vi "Comic Manager.vi"() -> ()   [LabVIEW 2024]
uses:
  TypeDefs/comic--cluster.ctl
  TypeDefs/series--cluster.ctl
  <userlib>/_OpenG.lib/file/file.llb/Strip Path Extension - String__ogtk.vi
  <userlib>/_OpenG.lib/file/file.llb/Strip Path Extension - Path__ogtk.vi
  <userlib>/_OpenG.lib/array/array.llb/Remove Duplicates from 1D Array (DBL)__ogtk.vi
  <userlib>/_OpenG.lib/array/array.llb/Sort 1D Array (String)__ogtk.vi
  <userlib>/_OpenG.lib/array/array.llb/openg_array.lvlib
  <userlib>/_OpenG.lib/file/file.llb/openg_file.lvlib
  <vilib>/httpClient/LabVIEWHTTPClient.lvlib
  <vilib>/addons/_JKI.lib/Serialization/JSON/JKI JSON Serialization.lvlib
panel:
  out "More Avail":bool
  out "Available?":bool
  in  "series tabs":enum32{"Add Issues", "Edit Series"}(tab)
  in  "New Issues":i32(listbox)
  out "new issue cover":picture
  in  "New Comics":path=path "D:/Comics/To Be Filed/Marvel"
  in  "move selected new":bool
  in  "move all new":bool
  in  "refresh":bool
  out "matching count":bool
  in  "comic info":T1
  in  "apply series changes":bool
  in  "series info":T2
  in  "Marvel Issues":i32(listbox)
  in  "launch renamer":bool
  in  "filter string":string
  in  "rename all cbz":bool
  in  "rename selected clz":bool
  in  "delete json issue":bool
  in  "rename json issue":bool
  out "synced":bool
  in  "create new folder":bool
  in  "json file path":path
  out "current details":i32(listbox)
  out "json details":i32(listbox)
  in  "launch cleaner":bool
  in  "Filter Current":bool
  out "json issue cover":picture
  out "current issue cover":picture
  in  "Series":i32(listbox)
  in  "Collected Issues":i32(listbox)
  in  "Folder":i32(listbox)
  in  "exit":bool
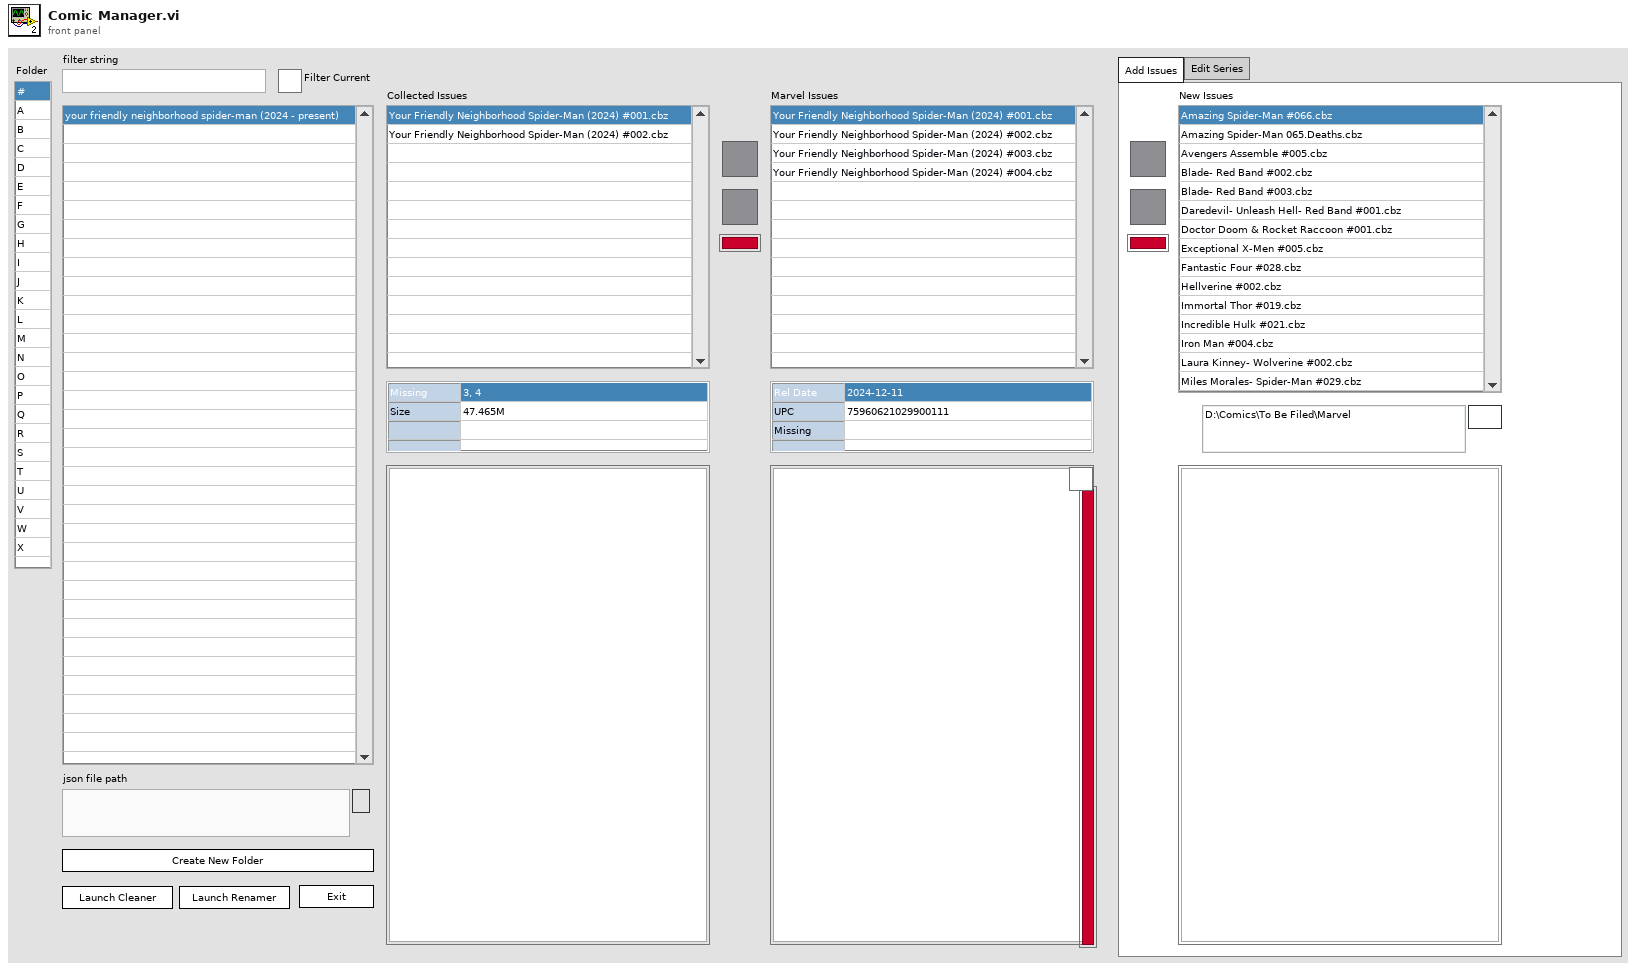
[diagram p1: front panel]
types:
  T1 = cluster{"rel date":string, "title":string, "description":string, "creators":string[], "characters":string[]}
  T2 = cluster{"seriesType":string, "title":string, "id":u32, "description":string, "start year":u32, "end year":u32, "tags":string[]}
  T3 = enum32{"Invalid", "Standard", "Closed", "Hidden", "Minimized", "Maximized"}
  T4 = enum32{"invalid app kind", "Development System", "Run Time System", "Student Edition", "Embedded LabVIEW", "Evaluation", "Custom"}
  T5 = enum16{"open", "replace", "create", "open or create", "replace or create", "replace or create with confirmation"}
  T6 = typedef "comic--cluster.ctl" = cluster{"id":i32, "digitalId":i32, "title":string, "issueNumber":i32, "variantDescription":string, "description":string, "modified":variant, "upc":string, "format":string, "pageCount":i32, "resourceURI":string, "urls":cluster{"type":string, "url":string}[], "series":cluster{"resourceURI":string, "name":string}, "dates":cluster{"type":string, "date":string}[], "prices":cluster{"price":dbl, "type":string}[], "thumbnail":cluster{"path":string, "extension":string}, "images":cluster{"path":string, "extension":string}[], "creators":cluster{"available":i32, "returned":i32, "collectionURI":string, "items":cluster{"resourceURI":string, "name":string, "role":string}[]}, "characters":cluster{"available":i32, "returned":i32, "collectionURI":string, "items":cluster{"resourceURI":string, "name":string}[]}, "stories":cluster{"available":i32, "returned":i32, "collectionURI":string, "items":cluster{"resourceURI":string, "name":string, "type":string}[]}, "events":cluster{"available":i32, "returned":i32, "collectionURI":string, "items":cluster{"resourceURI":string, "name":string}[]}}
  T7 = typedef "series--cluster.ctl" = cluster{"id":i32, "title":string, "description":string, "resourceURI":string, "urls":cluster{"type":string, "url":string}[], "startYear":i32, "endYear":i32, "rating":string, "type":string, "modified":variant, "thumbnail":cluster{"path":string, "extension":string}, "creators":cluster{"available":i32, "returned":i32, "collectionURI":string, "items":cluster{"resourceURI":string, "name":string, "role":string}[]}, "comics":cluster{"available":i32, "returned":i32, "collectionURI":string, "items":cluster{"resourceURI":string, "name":string}[]}, "characters":cluster{"available":i32, "returned":i32, "collectionURI":string, "items":cluster{"resourceURI":string, "name":string}[]}, "stories":cluster{"available":i32, "returned":i32, "collectionURI":string, "items":cluster{"resourceURI":string, "name":string, "type":string}[]}, "events":cluster{"available":i32, "returned":i32, "collectionURI":string, "items":cluster{"resourceURI":string, "name":string}[]}, "next":variant, "previous":variant, "tags":string[]}
  T8 = cluster{"Core":cluster{"Current VI Reference":refnum<vi>, "Close Panel on Exit?":bool}, "repo path":path, "series path":path, "json present":bool, "comic jsons":T6[], "local working folder":path, "display web":bool, "new working folder":path, "current missing":string, "json missing":string, "json dup":string, "current size":string, "web cover path":path, "series json":T7}
  T9 = cluster{"Current VI Reference":refnum<vi>, "Close Panel on Exit?":bool}
  T10 = typedef "comics.reply--cluster.ctl" = cluster{"code":i32, "status":string, "etag":string, "data":cluster{"offset":i32, "limit":i32, "total":i32, "count":i32, "results":T6[]}}
  T11 = typedef "imagedata.ctl" = cluster{"image type":i32, "image depth":i32, "image":u8[], "mask":u8[], "colors":u32[], "Rectangle":cluster{"left":i16, "top":i16, "right":i16, "bottom":i16}}
  T12 = typedef "LVBoundsTypeDef.ctl" = cluster{"Width":u32, "Height":u32}
  T13 = cluster{"resourceURI":string, "name":string, "role":string}[]
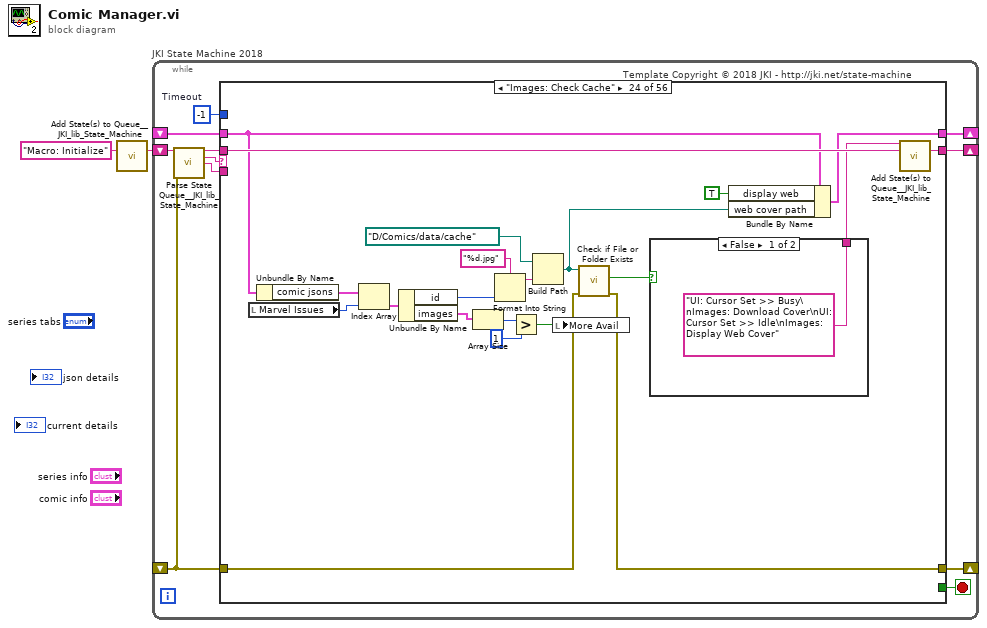
[diagram p0: block diagram]
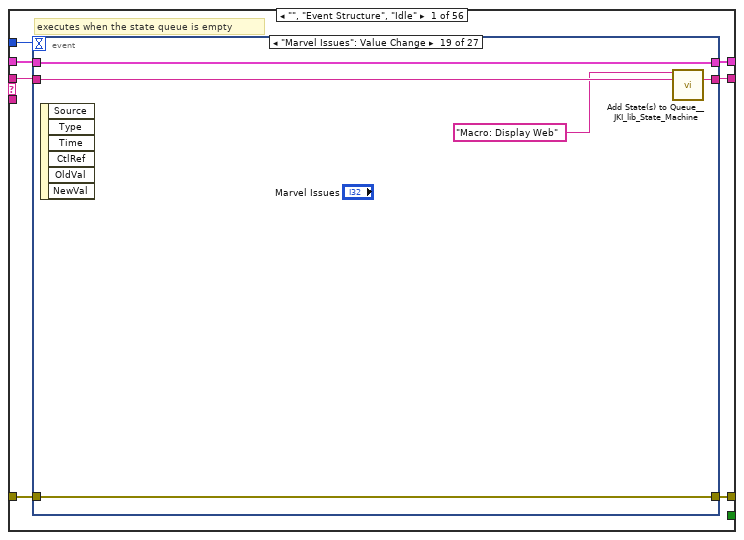
[diagram p2: hidden frame]
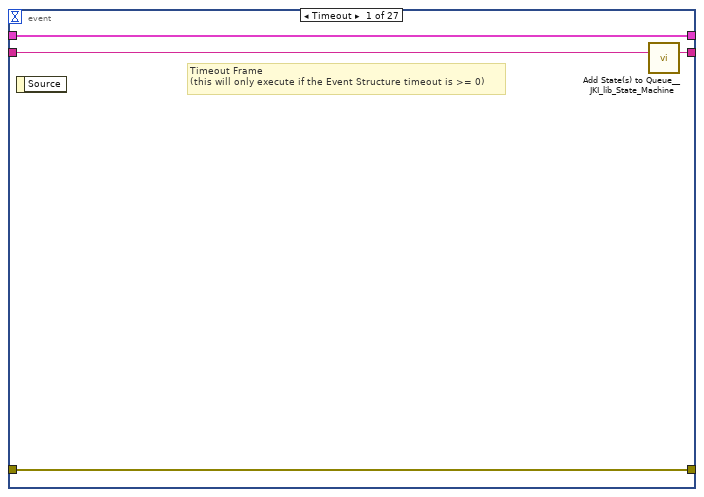
[diagram p3: hidden frame]
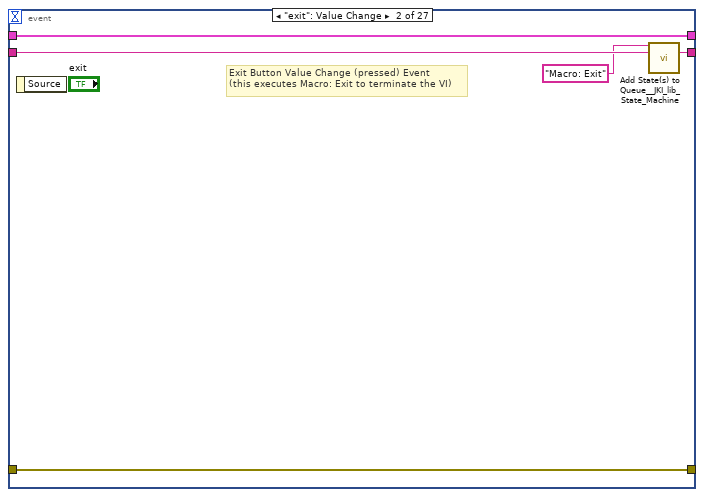
[diagram p4: hidden frame]
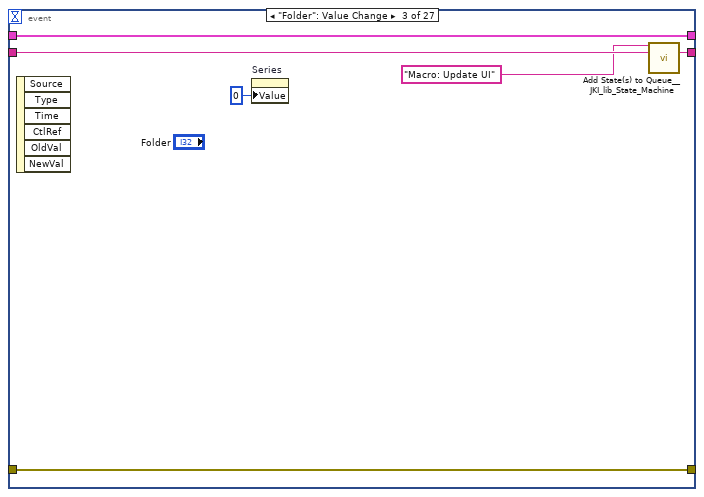
[diagram p5: hidden frame]
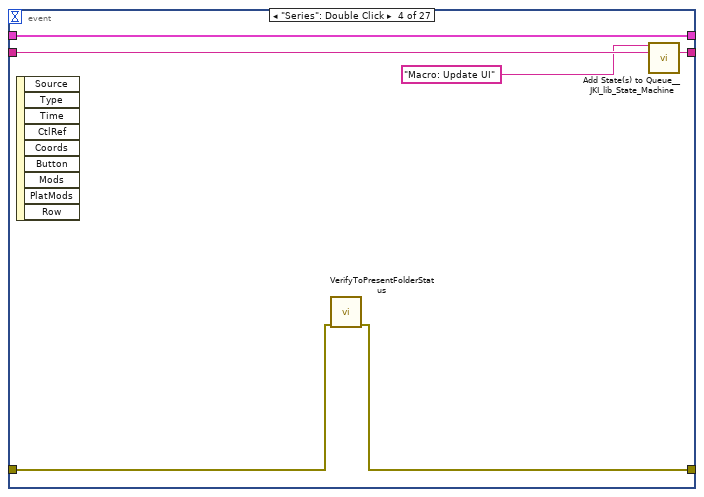
[diagram p6: hidden frame]
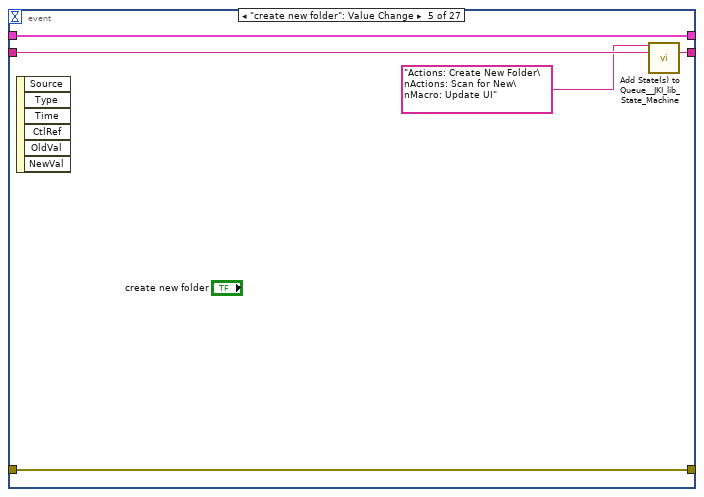
[diagram p7: hidden frame]
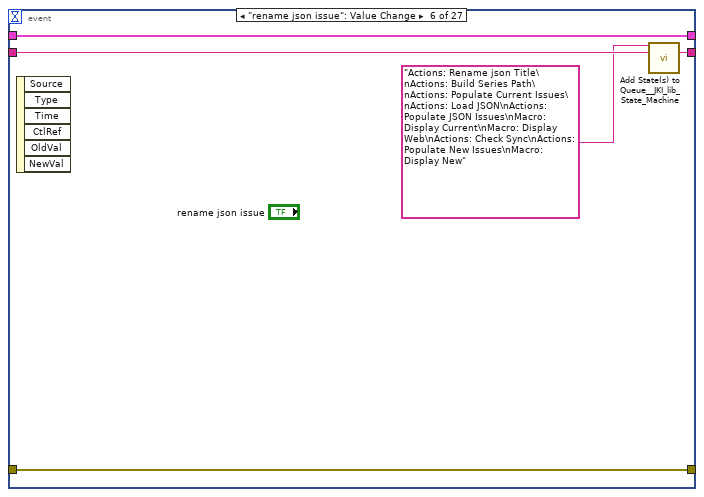
[diagram p8: hidden frame]
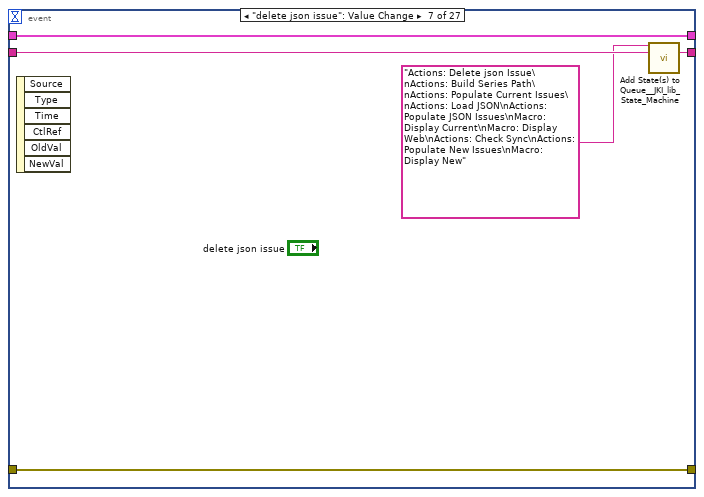
[diagram p9: hidden frame]
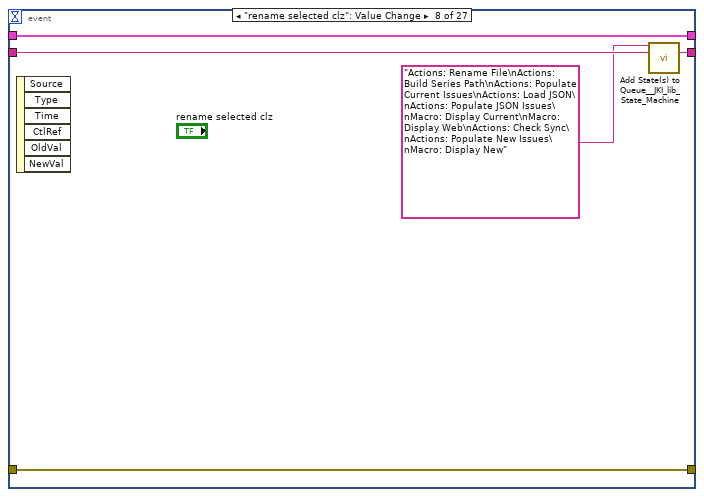
[diagram p10: hidden frame]
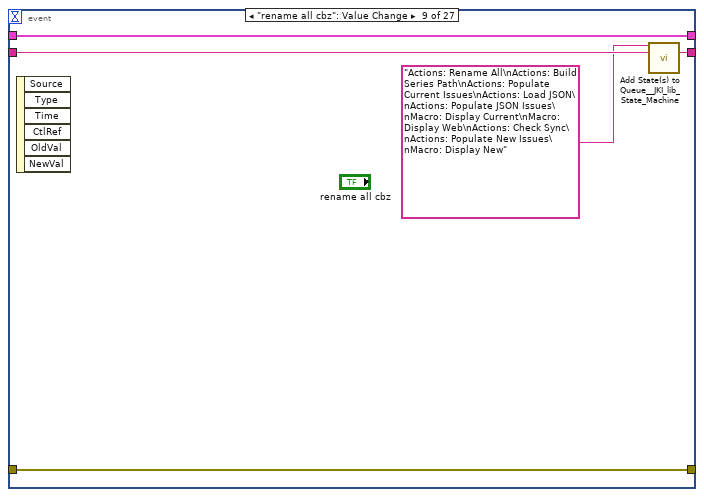
[diagram p11: hidden frame]
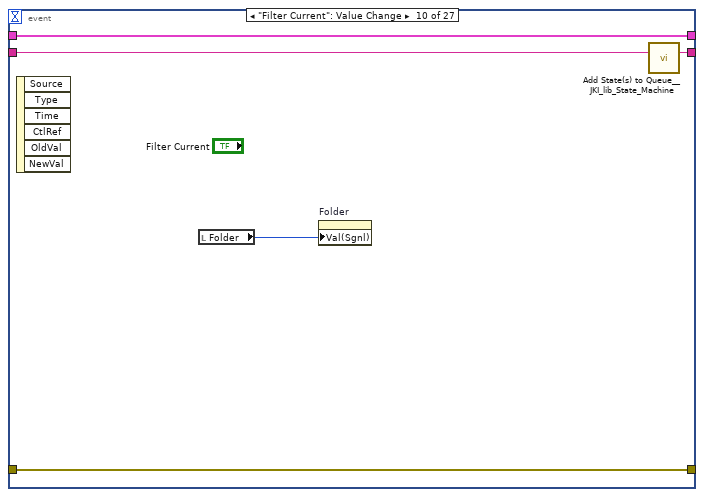
[diagram p12: hidden frame]
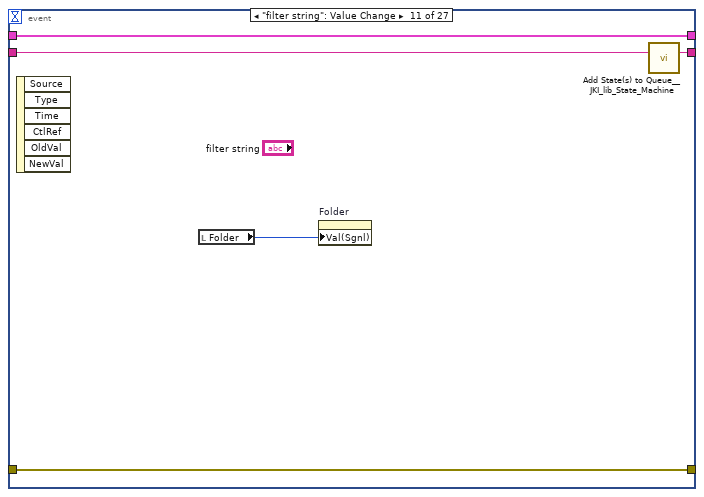
[diagram p13: hidden frame]
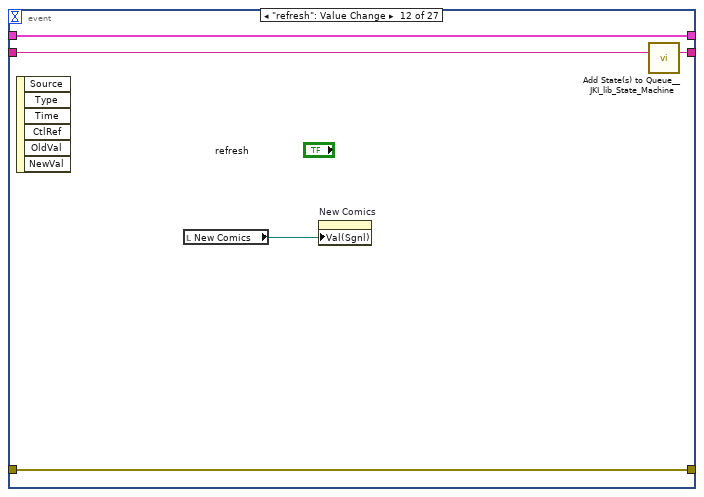
[diagram p14: hidden frame]
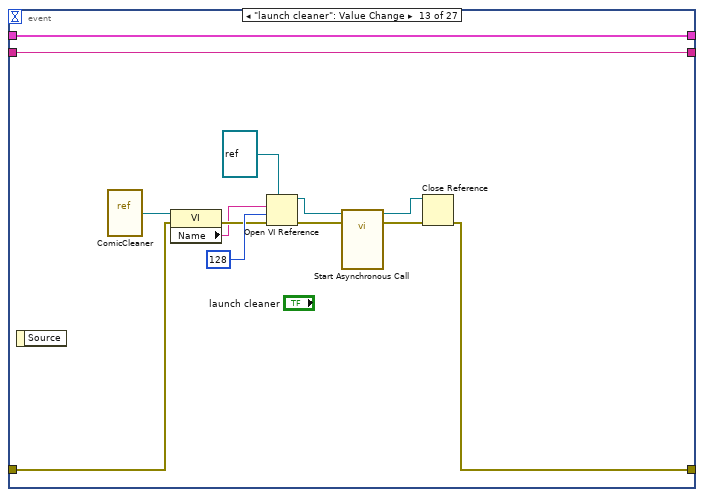
[diagram p15: hidden frame]
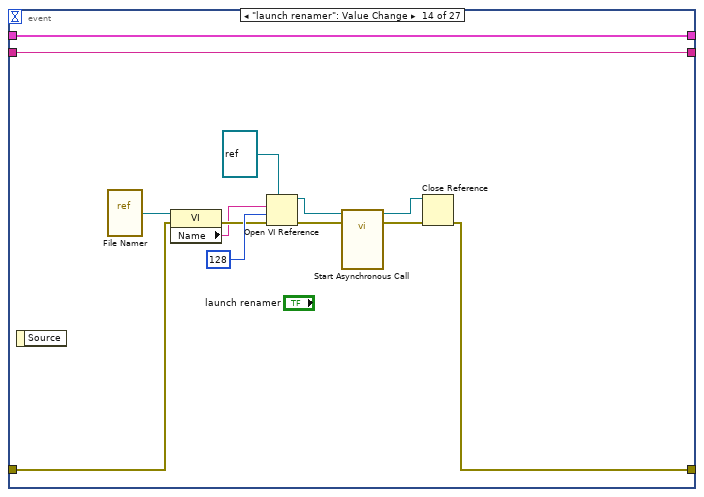
[diagram p16: hidden frame]
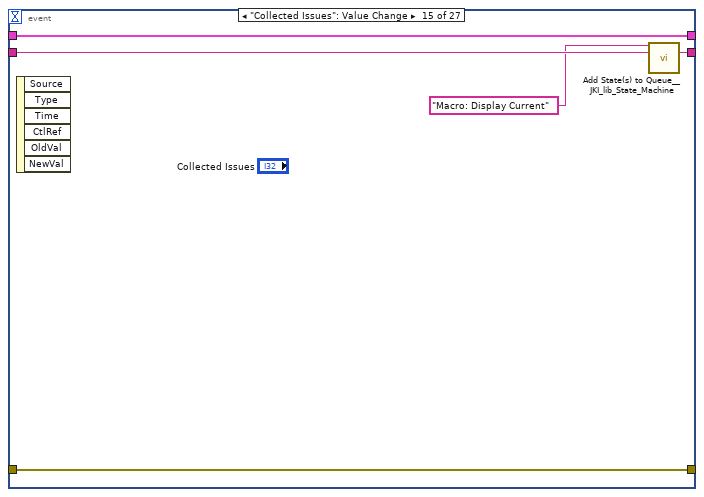
[diagram p17: hidden frame]
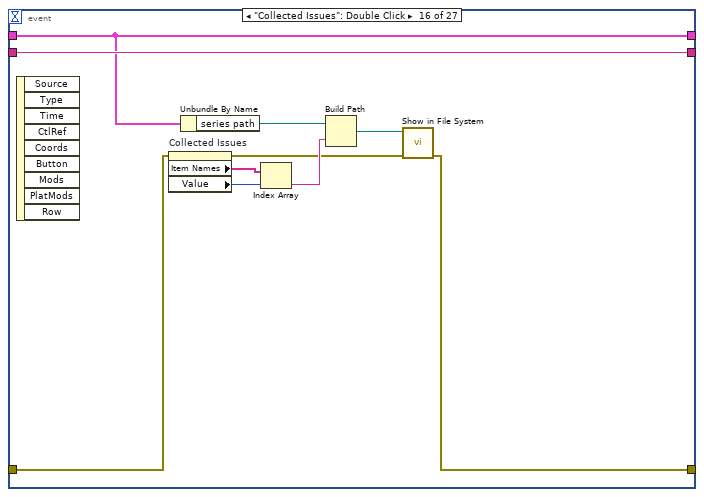
[diagram p18: hidden frame]
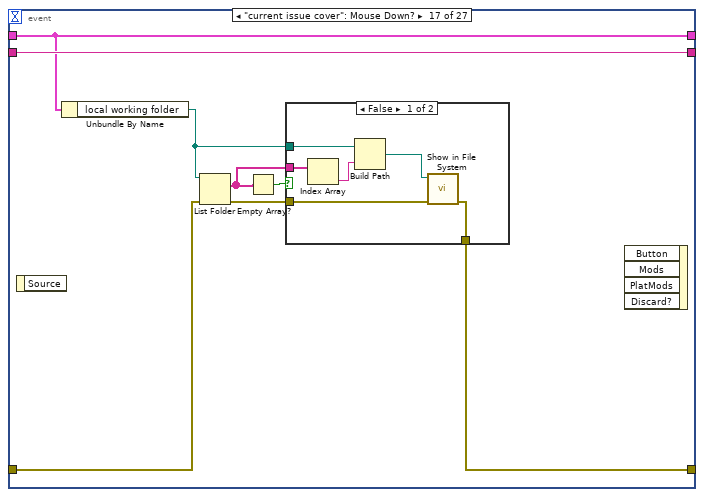
[diagram p19: hidden frame]
diagram:
  n1 = call <vilib>:"Add State(s) to Queue__JKI_lib_State_Machine.vi"("State(s) in (\"\")"="Macro: Initialize") -> ("States Out"=w2:string)  [unwired: 14 in]
  n2 = while "JKI State Machine 2018" {
    shift-right: [w6] -> _
    shift-left: _ -> [w5]
    shift-right: [w9] -> _
    shift-left: _ -> [w3]
    shift-right: [w8] -> _
    shift-left: w2 -> [w10]
    stop <- w7 stop-if-true
    w4 = -1  # Timeout
    # "Template Copyright © 2018 JKI - http://jki.net/state-machine"
    n3 = call <vilib>:"Parse State Queue__JKI_lib_State_Machine.vi"("State Queue"=w10, "Error In (no error)"=w3) -> ("Remaining States"=w12:string, "Current State"=w13:string, "Arguments"=w11:string)  [unwired: 11 in]
    n4 = case shown="\"Images: Check Cache\"" w13 {
      selector: w13 -> [_ _ w205 _ _ _ _ _ _ _ _ _ _ _ _ _ _ _ _ _ _ _ _ _ _ _ _ _ _ _ _ _ _ _ _ _ _ _ _ _ _ _ _ _ _ _ _ _ _ _ _ _ _ _ _ _]
      tunnel: w12 -> [w20 w204 w209 w228 w234 w239 w243 w261 w282 w300 w304 w314 w320 w331 w400 w405 w410 w415 w420 w425 w430 w440 w444 w465 w483 w514 w533 w562 w568 w592 w627 w651 w691 w727 w731 w748 w765 w792 w799 w821 w849 w857 w895 w930 w956 w979 w1016 w1034 w1064 w1082 w1108 w1135 w1145 w1155 w1165 w1210]
      tunnel: w11 -> [_ _ _ _ _ _ _ _ _ _ _ _ w315 w325 _ _ _ _ _ _ _ _ _ _ _ _ _ _ _ _ _ _ _ _ _ _ _ _ _ _ _ _ _ _ _ _ _ _ _ _ _ _ _ _ _ _]
      tunnel: w5 -> [w18 w201 w207 w221 w231 w237 w240 _ w272 w295 w301 w312 w318 w327 w397 w402 w407 w412 w417 w422 w427 w437 w441 w449 w471 w512 w523 w559 w565 w583 w618 w645 w682 w712 w728 w744 w762 w782 w797 w819 w847 w855 w893 w928 w954 w969 w1012 w1032 w1056 w1077 w1095 w1121 w1143 w1153 w1161 w1206]
      tunnel: [w17 w202 w211 w225 errorcluster {"status"=FALSE, "code"=0, "source"=""} ("error out") w236 w241 w258 w273 w296 w302 w306 w316 w328 w398 w403 w408 w413 w418 w423 w428 w438 w442 w455 w468 w488 w524 w558 w564 w569 w605 w649 w684 w711 w729 w741 w763 w766 w794 w816 w846 w851 w892 w925 w944 w961 w1006 w1031 w1049 w1074 w1100 w1123 w1137 w1148 w1157 w1182] -> w9
      tunnel: w3 -> [w16 w202 w210 w225 w230 w236 w241 w258 w266 w297 w302 w311 w317 w329 w398 w403 w408 w413 w418 w423 w428 w438 w442 w456 w473 w497 w525 w557 w563 w582 w617 w644 w683 w710 w729 w741 w763 w779 w795 w817 w845 w852 w889 w926 w945 w964 w995 w1030 w1050 w1075 w1102 w1124 w1141 w1152 w1158 w1208]
      tunnel: [w19 w203 w208 w227 w233 w238 w242 w260 w281 w299 w303 w313 w319 w330 w399 w404 w409 w414 w419 w424 w429 w439 w443 w464 w482 w513 w532 w561 w567 w591 w626 w650 w690 w726 w730 w747 w764 w791 w798 w820 w848 w856 w894 w929 w955 w978 w1015 w1033 w1063 w1081 w1107 w1134 w1144 w1154 w1164 w1209] -> w8
      tunnel: [_ _ _ _ _ TRUE _ _ _ _ _ _ _ _ _ _ _ _ _ _ _ _ _ _ _ _ _ _ _ _ _ _ _ _ _ _ _ _ _ _ _ _ _ _ _ _ _ _ _ _ _ _ _ _ _ _] -> w7
      tunnel: [w15 w201 w207 w226 w231 w237 w240 w259 w271 w295 w301 w312 w318 w327 w397 w402 w407 w412 w417 w422 w427 w437 w441 w451 w471 w511 w522 w559 w565 w583 w618 w645 w680 w712 w728 w744 w762 w781 w797 w819 w847 w850 w891 w928 w954 w965 w1012 w1032 w1056 w1077 w1095 w1120 w1143 w1153 w1160 w1205] -> w6
      tunnel: w4 -> [w14 _ _ _ _ _ _ _ _ _ _ _ _ _ _ _ _ _ _ _ _ _ _ _ _ _ _ _ _ _ _ _ _ _ _ _ _ _ _ _ _ _ _ _ _ _ _ _ _ _ _ _ _ _ _ _]
      frame "", "Event Structure", "Idle" {
        # "executes when the state queue is empty"
        n5 = event shown="[18] \"Marvel Issues\": Value Change" {
          selector: _ -> [_ _ _ _ _ _ _ _ _ _ _ _ _ _ _ _ _ _ _ _ _ _ _ _ _ _ _]
          dyn-events: _ -> [_ _ _ _ _ _ _ _ _ _ _ _ _ _ _ _ _ _ _ _ _ _ _ _ _ _ _]
          timeout: w14 -> [_ _ _ _ _ _ _ _ _ _ _ _ _ _ _ _ _ _ _ _ _ _ _ _ _ _ _]
          tunnel: w20 -> [w24 w29 w35 w41 w46 w51 w56 w61 w66 w71 w76 w81 w93 w106 w112 w122 w130 w144 w157 w161 w169 w174 w179 w184 w188 w194 w200]
          tunnel: [w23 w28 w34 w40 w45 w50 w55 w60 w65 w70 w75 w80 w93 w106 w111 w122 w130 w144 w156 w163 w168 w173 w178 w183 w186 w193 w199] -> w19
          tunnel: w18 -> [w21 w26 w32 w39 w43 w48 w53 w58 w63 w68 w73 w78 w94 w107 w109 w121 w129 w145 w154 w160 w166 w171 w176 w182 w189 w191 w197]
          tunnel: [w22 w27 w33 w36 w44 w49 w54 w59 w64 w69 w74 w79 w87 w100 w110 w114 w125 w140 w155 w159 w167 w172 w177 w181 w185 w190 w198] -> w17
          tunnel: w16 -> [w22 w27 w33 w37 w44 w49 w54 w59 w64 w69 w74 w79 w86 w99 w110 w115 w127 w143 w155 w159 w167 w172 w177 w181 w185 w190 w198]
          tunnel: [w21 w26 w32 w39 w43 w48 w53 w58 w63 w68 w73 w78 w94 w107 w109 w121 w129 w145 w154 w160 w166 w171 w176 w182 w189 w191 w197] -> w15
          event Timeout {
            # "Timeout Frame\n(this will only execute if the Event Structure timeout is >= 0)"
            n6 = event-data() -> ()  [unwired: 1 in, 1 out]
            n7 = call <vilib>:"Add State(s) to Queue__JKI_lib_State_Machine.vi"("State(s) in (\"\")"=w24) -> ("States Out"=w23:string)  [unwired: 14 in]
          }
          event "exit": Value Change {
            # "Exit Button Value Change (pressed) Event\n(this executes Macro: Exit to terminate the VI)"
            n8 = event-data() -> ()  [unwired: 1 in, 1 out]
            n9 = call <vilib>:"Add State(s) to Queue__JKI_lib_State_Machine.vi"("State(s) in Front (\"\")"="Macro: Exit", "State(s) in (\"\")"=w29) -> ("States Out"=w28:string)  [unwired: 13 in]
          }
          event "Folder": Value Change {
            n10 = event-data() -> ()  [unwired: 1 in, 6 out]
            n11 = property on="Series" class="LstBox (strict)"("Value"=0 ("Series")) -> ()  [unwired: 2 in, 2 out]
            n12 = call <vilib>:"Add State(s) to Queue__JKI_lib_State_Machine.vi"("State(s) in Front (\"\")"="Macro: Update UI", "State(s) in (\"\")"=w35) -> ("States Out"=w34:string)  [unwired: 13 in]
          }
          event "Series": Double Click {
            n13 = event-data() -> ()  [unwired: 1 in, 9 out]
            n14 = call "VerifyToPresentFolderStatus.vi"("error in (no error)"=w37) -> ("error out"=w36:errorcluster)  [unwired: 9 in, 1 out]
            n15 = call <vilib>:"Add State(s) to Queue__JKI_lib_State_Machine.vi"("State(s) in Front (\"\")"="Macro: Update UI", "State(s) in (\"\")"=w41) -> ("States Out"=w40:string)  [unwired: 13 in]
          }
          event "create new folder": Value Change {
            n16 = event-data() -> ()  [unwired: 1 in, 6 out]
            n17 = call <vilib>:"Add State(s) to Queue__JKI_lib_State_Machine.vi"("State(s) in Front (\"\")"="Actions: Create New Folder\nActions: Scan for New\nMacro: Update UI", "State(s) in (\"\")"=w46) -> ("States Out"=w45:string)  [unwired: 13 in]
          }
          event "rename json issue": Value Change {
            n18 = event-data() -> ()  [unwired: 1 in, 6 out]
            n19 = call <vilib>:"Add State(s) to Queue__JKI_lib_State_Machine.vi"("State(s) in Front (\"\")"="Actions: Rename json Title\nActions: Build Series Path\nActions: Populate Current Issues\nActions: Load JSON\nActions: Populate JSON Issues\nMacro: Display Current\nMacro: Display Web\nActions: Check Sync\nActions: Populate New Issues\nMacro: Display New", "State(s) in (\"\")"=w51) -> ("States Out"=w50:string)  [unwired: 13 in]
          }
          event "delete json issue": Value Change {
            n20 = event-data() -> ()  [unwired: 1 in, 6 out]
            n21 = call <vilib>:"Add State(s) to Queue__JKI_lib_State_Machine.vi"("State(s) in Front (\"\")"="Actions: Delete json Issue\nActions: Build Series Path\nActions: Populate Current Issues\nActions: Load JSON\nActions: Populate JSON Issues\nMacro: Display Current\nMacro: Display Web\nActions: Check Sync\nActions: Populate New Issues\nMacro: Display New", "State(s) in (\"\")"=w56) -> ("States Out"=w55:string)  [unwired: 13 in]
          }
          event "rename selected clz": Value Change {
            n22 = event-data() -> ()  [unwired: 1 in, 6 out]
            n23 = call <vilib>:"Add State(s) to Queue__JKI_lib_State_Machine.vi"("State(s) in Front (\"\")"="Actions: Rename File\nActions: Build Series Path\nActions: Populate Current Issues\nActions: Load JSON\nActions: Populate JSON Issues\nMacro: Display Current\nMacro: Display Web\nActions: Check Sync\nActions: Populate New Issues\nMacro: Display New", "State(s) in (\"\")"=w61) -> ("States Out"=w60:string)  [unwired: 13 in]
          }
          event "rename all cbz": Value Change {
            n24 = event-data() -> ()  [unwired: 1 in, 6 out]
            n25 = call <vilib>:"Add State(s) to Queue__JKI_lib_State_Machine.vi"("State(s) in Front (\"\")"="Actions: Rename All\nActions: Build Series Path\nActions: Populate Current Issues\nActions: Load JSON\nActions: Populate JSON Issues\nMacro: Display Current\nMacro: Display Web\nActions: Check Sync\nActions: Populate New Issues\nMacro: Display New", "State(s) in (\"\")"=w66) -> ("States Out"=w65:string)  [unwired: 13 in]
          }
          event "Filter Current": Value Change {
            n26 = event-data() -> ()  [unwired: 1 in, 6 out]
            n27 = local read "Folder"() -> (w67:i32)
            n28 = property on="Folder" class="LstBox (strict)"("Val(Sgnl)"=w67) -> ()  [unwired: 2 in, 2 out]
            n29 = call <vilib>:"Add State(s) to Queue__JKI_lib_State_Machine.vi"("State(s) in (\"\")"=w71) -> ("States Out"=w70:string)  [unwired: 14 in]
          }
          event "filter string": Value Change {
            n30 = event-data() -> ()  [unwired: 1 in, 6 out]
            n31 = local read "Folder"() -> (w72:i32)
            n32 = property on="Folder" class="LstBox (strict)"("Val(Sgnl)"=w72) -> ()  [unwired: 2 in, 2 out]
            n33 = call <vilib>:"Add State(s) to Queue__JKI_lib_State_Machine.vi"("State(s) in (\"\")"=w76) -> ("States Out"=w75:string)  [unwired: 14 in]
          }
          event "refresh": Value Change {
            n34 = event-data() -> ()  [unwired: 1 in, 6 out]
            n35 = local read "New Comics"() -> (w77:path)
            n36 = property on="New Comics" class="Path"("Val(Sgnl)"=w77) -> ()  [unwired: 2 in, 2 out]
            n37 = call <vilib>:"Add State(s) to Queue__JKI_lib_State_Machine.vi"("State(s) in (\"\")"=w81) -> ("States Out"=w80:string)  [unwired: 14 in]
          }
          event "launch cleaner": Value Change {
            n38 = event-data() -> ()  [unwired: 1 in, 1 out]
            n39 = vi-ref "ComicCleaner.vi"() -> (w91:refnum<vi>)
            n40 = property class="VI"(reference=w91, error in=w86) -> (error out=w90:errorcluster, "Name"=w89:string)  [unwired: 1 out]
            n41 = Open VI Reference(type specifier VI Refnum (for type only)=refnum<vi> refnum, vi path=w89, options=128, error in (no error)=w90) -> (vi reference=w85:refnum<vi>, error out=w83:errorcluster)  [unwired: 2 in]
            n42 = call-by-ref "Start Asynchronous Call"(reference=w85, error in=w83) -> (reference out=w84:refnum<vi>, error out=w82:errorcluster)  [unwired: 12 in]
            n43 = Close Reference(reference=w84, error in (no error)=w82) -> (error out=w87:errorcluster)
          }
          event "launch renamer": Value Change {
            n44 = event-data() -> ()  [unwired: 1 in, 1 out]
            n45 = vi-ref "File Namer.vi"() -> (w104:refnum<vi>)
            n46 = property class="VI"(reference=w104, error in=w99) -> (error out=w103:errorcluster, "Name"=w102:string)  [unwired: 1 out]
            n47 = Open VI Reference(type specifier VI Refnum (for type only)=refnum<vi> refnum, vi path=w102, options=128, error in (no error)=w103) -> (vi reference=w98:refnum<vi>, error out=w96:errorcluster)  [unwired: 2 in]
            n48 = call-by-ref "Start Asynchronous Call"(reference=w98, error in=w96) -> (reference out=w97:refnum<vi>, error out=w95:errorcluster)  [unwired: 12 in]
            n49 = Close Reference(reference=w97, error in (no error)=w95) -> (error out=w100:errorcluster)
          }
          event "Collected Issues": Value Change {
            n50 = event-data() -> ()  [unwired: 1 in, 6 out]
            n51 = call <vilib>:"Add State(s) to Queue__JKI_lib_State_Machine.vi"("State(s) in Front (\"\")"="Macro: Display Current", "State(s) in (\"\")"=w112) -> ("States Out"=w111:string)  [unwired: 13 in]
          }
          event "Collected Issues": Double Click {
            n52 = event-data() -> ()  [unwired: 1 in, 9 out]
            n53 = property on="Collected Issues" class="LstBox (strict)"(error in=w115) -> (error out=w116:errorcluster, "Item Names"=w120:string[], "Value"=w119:i32)  [unwired: 1 in, 1 out]
            n54 = Unbundle By Name(w121) -> ("series path"=w117:path)
            n55 = Index Array(array=w120, index=w119) -> (element=w118:string)
            n56 = Build Path(base path=w117, name or relative path=w118) -> (appended path=w113:path)
            n57 = call <vilib>:"Show in File System.vi"("error in (no error)"=w116, "file or directory path"=w113) -> ("error out"=w114:errorcluster)  [unwired: 9 in]
          }
          event "current issue cover": Mouse Down? {
            n58 = event-data() -> ()  [unwired: 1 in, 1 out]
            n59 = Unbundle By Name(w129) -> ("local working folder"=w128:path)
            n60 = List Folder(path=w128, error in=w127) -> (filenames=w124:string[], error out=w126:errorcluster)  [unwired: 2 in, 2 out]
            n61 = Empty Array?(array=w124) -> (empty?=w123:bool)
            n62 = case shown="False" w123 {
              tunnel: w128 -> [w135 _]
              tunnel: w126 -> [w134 w137]
              tunnel: [w132 w137] -> w125
              tunnel: w124 -> [w131 _]
              frame False {
                n63 = Index Array(array=w131) -> (element=w136:string)  [unwired: 1 in]
                n64 = Build Path(base path=w135, name or relative path=w136) -> (appended path=w133:path)
                n65 = call <vilib>:"Show in File System.vi"("error in (no error)"=w134, "file or directory path"=w133) -> ("error out"=w132:errorcluster)  [unwired: 9 in]
              }
              frame True {
              }
            }
            n66 = event-data() -> ()  [unwired: 5 in, 1 out]
          }
          event "new issue cover": Mouse Down? {
            n67 = event-data() -> ()  [unwired: 1 in, 8 out]
            n68 = Unbundle By Name(w145) -> ("new working folder"=w142:path)
            n69 = List Folder(path=w142, error in=w143) -> (filenames=w138:string[], error out=w141:errorcluster)  [unwired: 2 in, 2 out]
            n70 = Empty Array?(array=w138) -> (empty?=w139:bool)
            n71 = case shown="True" w139 {
              tunnel: w138 -> [w150 _]
              tunnel: w142 -> [w149 _]
              tunnel: w141 -> [w148 w152]
              tunnel: [w146 w152] -> w140
              frame False {
                n72 = Index Array(array=w150) -> (element=w151:string)  [unwired: 1 in]
                n73 = Build Path(base path=w149, name or relative path=w151) -> (appended path=w147:path)
                n74 = call <vilib>:"Show in File System.vi"("error in (no error)"=w148, "file or directory path"=w147) -> ("error out"=w146:errorcluster)  [unwired: 9 in]
              }
              frame True {
              }
            }
            n75 = event-data() -> ()  [unwired: 5 in, 1 out]
          }
          event "Marvel Issues": Value Change {
            n76 = event-data() -> ()  [unwired: 1 in, 6 out]
            n77 = call <vilib>:"Add State(s) to Queue__JKI_lib_State_Machine.vi"("State(s) in Front (\"\")"="Macro: Display Web", "State(s) in (\"\")"=w157) -> ("States Out"=w156:string)  [unwired: 13 in]
          }
          event "json issue cover": Mouse Down? {
            n78 = event-data() -> ()  [unwired: 1 in, 1 out]
            n79 = local read "More Avail"() -> (w158:bool)
            n80 = case shown="True" w158 {
              tunnel: [_ "Images: Rotate json Image\nImages: Remove from Cache\nMacro: Display Web"] -> w162
              frame False {
              }
              frame True {
              }
            }
            n81 = event-data() -> ()  [unwired: 5 in, 1 out]
            n82 = call <vilib>:"Add State(s) to Queue__JKI_lib_State_Machine.vi"("State(s) in Front (\"\")"=w162, "State(s) in (\"\")"=w161) -> ("States Out"=w163:string)  [unwired: 13 in]
          }
          event "New Issues": Value Change {
            n83 = event-data() -> ()  [unwired: 1 in, 6 out]
            n84 = call <vilib>:"Add State(s) to Queue__JKI_lib_State_Machine.vi"("State(s) in Front (\"\")"="Macro: Display New", "State(s) in (\"\")"=w169) -> ("States Out"=w168:string)  [unwired: 13 in]
          }
          event "move selected new": Value Change {
            n85 = event-data() -> ()  [unwired: 1 in, 6 out]
            n86 = call <vilib>:"Add State(s) to Queue__JKI_lib_State_Machine.vi"("State(s) in Front (\"\")"="Actions: Move Selected\nActions: Build Series Path\nActions: Populate Current Issues\nActions: Load JSON\nActions: Populate JSON Issues\nMacro: Display Current\nMacro: Display Web\nActions: Check Sync\nActions: Populate New Issues\nMacro: Display New", "State(s) in (\"\")"=w174) -> ("States Out"=w173:string)  [unwired: 13 in]
          }
          event "move all new": Value Change {
            n87 = event-data() -> ()  [unwired: 1 in, 6 out]
            n88 = call <vilib>:"Add State(s) to Queue__JKI_lib_State_Machine.vi"("State(s) in Front (\"\")"="Actions: Move All\nActions: Build Series Path\nActions: Populate Current Issues\nActions: Load JSON\nActions: Populate JSON Issues\nMacro: Display Current\nMacro: Display Web\nActions: Check Sync\nActions: Populate New Issues\nMacro: Display New", "State(s) in (\"\")"=w179) -> ("States Out"=w178:string)  [unwired: 13 in]
          }
          event "Series": Value Change {
            n89 = event-data() -> ()  [unwired: 1 in, 1 out]
            n90 = call <vilib>:"Add State(s) to Queue__JKI_lib_State_Machine.vi"("State(s) in Front (\"\")"="Actions: Build Series Path\nActions: Populate Current Issues\nActions: Load JSON\nActions: Populate JSON Issues\nMacro: Display Current\nMacro: Display Web\nActions: Check Sync\nActions: Populate New Issues\nActions: Populate Series Info\nMacro: Display New", "State(s) in (\"\")"=w184) -> ("States Out"=w183:string)  [unwired: 13 in]
          }
          event "apply series changes": Value Change {
            n91 = event-data() -> ()  [unwired: 1 in, 6 out]
            n92 = call <vilib>:"Add State(s) to Queue__JKI_lib_State_Machine.vi"("State(s) in Front (\"\")"="Actions: Apply Series Changes", "State(s) in (\"\")"=w188) -> ("States Out"=w186:string)  [unwired: 13 in]
          }
          event "New Comics": Value Change {
            n93 = event-data() -> ()  [unwired: 1 in, 6 out]
            n94 = call <vilib>:"Add State(s) to Queue__JKI_lib_State_Machine.vi"("State(s) in Front (\"\")"="Actions: Populate New Issues\nMacro: Display New", "State(s) in (\"\")"=w194) -> ("States Out"=w193:string)  [unwired: 13 in]
          }
          event Panel Close? {
            # "Discard the event because we'll close the front panel ourselves in Macro: Exit"
            # "Close Panel button (pressed) Event\n(this executes Macro: Exit to terminate the VI)"
            n95 = event-data() -> ()  [unwired: 1 in, 1 out]
            n96 = event-data("Discard?"=TRUE) -> ()  [unwired: 1 in, 1 out]
            n97 = call <vilib>:"Add State(s) to Queue__JKI_lib_State_Machine.vi"("State(s) in Front (\"\")"="Macro: Exit", "State(s) in (\"\")"=w200) -> ("States Out"=w199:string)  [unwired: 13 in]
          }
        }
      }
      frame "---------- Core ----------" {
        # "Do not put any code in this frame.\n(it is a separator no-op)"
        n98 = call <vilib>:"Add State(s) to Queue__JKI_lib_State_Machine.vi"("State(s) in (\"\")"=w204) -> ("States Out"=w203:string)  [unwired: 14 in]
      }
      frame Default {
        w214 = 42 items=["No error", "Argument error", "Memory is full", "Out of zone", "End of file", "File already open", "Generic file I/O error", "File not found", "File permission error", "Disk is full", "Duplicate path", "Too many files open", "System feature not enabled", "Resource file not found", "Cannot add resource", "Resource not found", "Image not found", "Image memory error", "Pen does not exist", "Config type invalid", "Config token not found", "Config parse error", "Config memory error", "Bad external code format", "Bad external code offset", "External code not present", "Null window", "Destroy window error", "Null menu", "Print aborted", "Bad print record", "Print driver error", "Windows error during printing", "Memory error during printing", "Print dialog error", "Generic print error", "Invalid device refnum", "Device not found", "Device parameter error", "Device unit error", "Cannot open device", "Device call aborted", "Generic error", "Cancelled by user", "Object ID too low", "Object ID too high", "Object not in heap", "Unknown heap", "Unknown object (invalid DefProc)", "Unknown object (DefProc not in table)", "Message out of range", "Invalid (null) method", "Unknown message", "Manager call not supported", "Bad address", "Network operation in progress", "Network operation timed out", "Connection is busy", "Network attribute not supported", "Network error", "Address in use", "System out of memory", "Connection aborted", "Connection refused", "Not connected", "Already connected", "Connection closed", "Initialization error (interapplication manager)", "Bad occurrence", "Wait on unbound occurrence handler", "Occurrence queue overflow", "Datalog type conflict", "Unused", "Unrecognized type (interapplication manager)", "Memory corrupt", "Failed to make temporary DLL", "Old CIN version", "Drag socket not found", "Failed to load drop-object", "Failed to register OLE object", "Failed to release OLE object", "Format specifier type mismatch", "Unknown format specifier", "Too few format specifiers", "Too many format specifiers", "Scan failed", "Newer CIN version", "Error converting to variant", "Runtime menu error", "Password tampered", "Variant attribute not found", "Incompatible variant data type", "Event data is not available", "Event Store is not present", "Occurrence is not found", "Event Queue is not created", "Event info is not available", "Refnum passed is NULL", "Error retrieving Class GUID", "Error retrieving CoClass GUID", "Error retrieving TypeLib GUID.", "Bad built application magic bytes.", "Specific driver is different from the specific driver associated with the Logical Name.", "There is no session opened to the class driver.", "Max Error", "MAX - Error with config objects", "MAX - Error loading configuration", "MAX - Group not supported"]
        # "Current State"
        # "Do not delete, rename, or modify this frame.\n(this is used to capture unhandled states and typos)"
        # "Handle mistyped state name (developer tool)"
        n99 = Format Into String(format string="Software Exception: Unhandled State \"%s\"." ("message"), error in=w210, w205) -> (resulting string=w213:string, error out=w212:errorcluster)  [unwired: 1 in]
        n100 = call <vilib>:"Error Cluster From Error Code.vi"("show call chain? (False)"=TRUE, "error in (no error)"=w212, "error message (\"\")"=w213, "error code (0)"=w214) -> ("error out"=w211:errorcluster)  [unwired: 5 in]
        n101 = call <vilib>:"Add State(s) to Queue__JKI_lib_State_Machine.vi"("State(s) in (\"\")"=w209) -> ("States Out"=w208:string)  [unwired: 14 in]
      }
      frame "Initialize Core Data" {
        # "Do not delete, rename, or modify this frame.\n(this is used to determine panel behavior on exit)"
        # "originally closed?"
        # "exe?"
        # "If panel starts closed or is an EXE, then close it when we exit"
        n102 = property class="VI"() -> ("FP.State"=w218:T3)  [unwired: 2 in, 2 out]
        n103 = property class="App"() -> ("App.Kind"=w224:T4)  [unwired: 2 in, 2 out]
        n104 = control-ref of="Current VI Reference"() -> (w219:refnum<vi>)
        n105 = Equal?(x=w218, y=T3."Closed" ("Front Panel Window:State")) -> (x = y?=w216:bool)
        n106 = Equal?(x=w224, y=T4."Run Time System" ("Application:Kind")) -> (x = y?=w222:bool)
        n107 = Or(x=w216, y=w222) -> (x .or. y?=w220:bool)
        n108 = Bundle By Name(cluster=w221, "Core.Current VI Reference"=w219, "Core.Close Panel on Exit?"=w220) -> (w226:T8)
        n109 = call <vilib>:"Add State(s) to Queue__JKI_lib_State_Machine.vi"("State(s) in (\"\")"=w228) -> ("States Out"=w227:string)  [unwired: 14 in]
      }
      frame "Error Handler" {
        # "Unhandled Error -- Display it"
        # "Handle any errors here.\nYou can also output any states to clean-up after errors occur"
        # "Clear error"
        n110 = call <vilib>:"General Error Handler.vi"("error in (no error)"=w230) -> ()  [unwired: 10 in, 5 out]
        n111 = call <vilib>:"Add State(s) to Queue__JKI_lib_State_Machine.vi"("State(s) in Front (\"\")"="/* Post Error States", "State(s) in (\"\")"=w234) -> ("States Out"=w233:string)  [unwired: 13 in]
      }
      frame "Exit" {
        # "Do not put any code in this frame.\n(No errors that occur here will be handled.)"
        n112 = call <vilib>:"Add State(s) to Queue__JKI_lib_State_Machine.vi"("State(s) in (\"\")"=w239) -> ("States Out"=w238:string)  [unwired: 14 in]
      }
      frame "---------- Data ----------" {
        # "Do not put any code in this frame.\n(It is a separator no-op. You can make a copy of this frame to create a new Data frame)"
        n113 = call <vilib>:"Add State(s) to Queue__JKI_lib_State_Machine.vi"("State(s) in (\"\")"=w243) -> ("States Out"=w242:string)  [unwired: 14 in]
      }
      frame "Data: Initialize" {
        w244 = T7 {"id"=0, "title"="", "description"="", "resourceURI"="", "urls"=[], "startYear"=0, "endYear"=0, "rating"="", "type"="", "modified"=variant, "thumbnail"={"path"="", "extension"=""}, "creators"={"available"=0, "returned"=0, "collectionURI"="", "items"=[]}, "comics"={"available"=0, "returned"=0, "collectionURI"="", "items"=[]}, "characters"={"available"=0, "returned"=0, "collectionURI"="", "items"=[]}, "stories"={"available"=0, "returned"=0, "collectionURI"="", "items"=[]}, "events"={"available"=0, "returned"=0, "collectionURI"="", "items"=[]}, "next"=variant, "previous"=variant, "tags"=[]}  # series json
        w245 = path "FileName_web"  # web cover path
        w246 = ""  # current size
        w247 = ""  # json dup
        w248 = ""  # json missing
        w249 = ""  # current missing
        w250 = path "FileName_new"  # new working folder
        w251 = TRUE  # display web
        w252 = path "FileName_local"  # local working folder
        w253 = T6[] []  # comic jsons
        w254 = TRUE  # json present
        w255 = path "D:/Comics/Marvel"  # series path
        w256 = T9 {"Current VI Reference"=refnum, "Close Panel on Exit?"=FALSE}  # Core
        w257 = path "D:/Comics/Marvel"  # repo path
        # "Initialize the shift-register data, here.\n(data names are defined by what you wire into the bundle function)"
        n114 = Bundle("Core"=w256, "repo path"=w257, "series path"=w255, "json present"=w254, "comic jsons"=w253, "local working folder"=w252, "display web"=w251, "new working folder"=w250, "current missing"=w249, "json missing"=w248, "json dup"=w247, "current size"=w246, "web cover path"=w245, "series json"=w244) -> (w259:T8)  [unwired: 1 in]
        n115 = call <vilib>:"Add State(s) to Queue__JKI_lib_State_Machine.vi"("State(s) in (\"\")"=w261) -> ("States Out"=w260:string)  [unwired: 14 in]
      }
      frame "Data: Init Temp Folders" {
        w264 = path "FileName_new"  # new working folder
        w280 = path "FileName_local"  # local working folder
        n116 = Temporary Directory() -> (w265:path)
        n117 = Build Path(base path=w265, name or relative path=w280) -> (appended path=w276:path)
        n118 = Build Path(base path=w265, name or relative path=w264) -> (appended path=w267:path)
        n119 = call <vilib>:"Check if File or Folder Exists.vi"("error in (no error)"=w266, "path"=w276) -> ("error out"=w279:errorcluster, "file or folder exists?"=w277:bool, "dup path"=w278:path)  [unwired: 7 in]
        n120 = call <vilib>:"Check if File or Folder Exists.vi"("error in (no error)"=w266, "path"=w267) -> ("error out"=w270:errorcluster, "file or folder exists?"=w268:bool, "dup path"=w269:path)  [unwired: 7 in]
        n121 = case shown="True" w277 {
          tunnel: w278 -> [w292 w294]
          tunnel: w279 -> [w291 w293]
          tunnel: [w290 w294] -> w275
          tunnel: [w289 w293] -> w274
          frame False {
            n122 = Create Folder(path (use dialog)=w292, error in=w291) -> (created path=w290:path, error out=w289:errorcluster)  [unwired: 1 in, 1 out]
          }
          frame True {
          }
        }
        n123 = case shown="True" w268 {
          tunnel: w269 -> [w286 w288]
          tunnel: w270 -> [w285 w287]
          tunnel: [w284 w288] -> w263
          tunnel: [w283 w287] -> w262
          frame False {
            n124 = Create Folder(path (use dialog)=w286, error in=w285) -> (created path=w284:path, error out=w283:errorcluster)  [unwired: 1 in, 1 out]
          }
          frame True {
          }
        }
        n125 = Merge Errors(w274, w262) -> (w273:errorcluster)
        n126 = Bundle By Name(cluster=w272, "local working folder"=w275, "new working folder"=w263) -> (w271:T8)
        n127 = call <vilib>:"Add State(s) to Queue__JKI_lib_State_Machine.vi"("State(s) in (\"\")"=w282) -> ("States Out"=w281:string)  [unwired: 14 in]
      }
      frame "Data: Cleanup" {
        # "Cleanup any data and references, here.\n(this is called automatically, by the Macro: Exit)"
        n128 = Unbundle By Name(w295) -> ("Core.Current VI Reference"=w298:refnum<vi>)
        n129 = Close Reference(reference=w298, error in (no error)=w297) -> (error out=w296:errorcluster)
        n130 = call <vilib>:"Add State(s) to Queue__JKI_lib_State_Machine.vi"("State(s) in (\"\")"=w300) -> ("States Out"=w299:string)  [unwired: 14 in]
      }
      frame "---------- UI ----------" {
        # "Do not put any code in this frame.\n(It is a separator no-op. You can make a copy of this frame to create a new UI frame)"
        n131 = call <vilib>:"Add State(s) to Queue__JKI_lib_State_Machine.vi"("State(s) in (\"\")"=w304) -> ("States Out"=w303:string)  [unwired: 14 in]
      }
      frame "UI: Initialize" {
        # "Initialize the User Interface, here.\n(this is called automatically, by the Macro: Init)"
        n132 = call "GenerateAlphabetArray.vi"() -> ("Array"=w309:string[])
        n133 = Build Array (concatenate)("#", w309) -> (w308:string[])
        n134 = property on="Folder" class="LstBox (strict)"(error in=w311, "Item Names"=w308) -> (error out=w307:errorcluster)  [unwired: 1 in, 1 out]
        n135 = property on="Collected Issues" class="LstBox (strict)"(error in=w307, "Value"=0 ("Current Issues")) -> (error out=w306:errorcluster)  [unwired: 1 in, 1 out]
        n136 = call <vilib>:"Add State(s) to Queue__JKI_lib_State_Machine.vi"("State(s) in (\"\")"=w314) -> ("States Out"=w313:string)  [unwired: 14 in]
      }
      frame "UI: Cursor Set" {
        # "Argument"
        # "Set and Unset Cursor Busy.\n(Usage: \"UI: Cursor Set >> Busy|Idle\")"
        n137 = case shown="\"Idle\", Default" w315 {
          tunnel: w317 -> [w322 w324]
          tunnel: [w321 w323] -> w316
          frame "Idle", Default {
            n138 = call <vilib>:"Unset Busy.vi"("error in (no error)"=w322) -> ("error out"=w321:errorcluster)  [unwired: 10 in]
          }
          frame "Busy" {
            n139 = call <vilib>:"Set Busy.vi"("error in (no error)"=w324) -> ("error out"=w323:errorcluster)  [unwired: 9 in, 1 out]
          }
        }
        n140 = call <vilib>:"Add State(s) to Queue__JKI_lib_State_Machine.vi"("State(s) in (\"\")"=w320) -> ("States Out"=w319:string)  [unwired: 14 in]
      }
      frame "UI: Front Panel State" {
        # "Argument"
        # "Set Front Panel Open or Closed\n(Usage: \"UI: Front Panel State >> Open|Close\")"
        n141 = Unbundle By Name(w327) -> ("Core.Current VI Reference"=w326:refnum<vi>)
        n142 = case shown="\"Open\", \"Standard\", Default" w325 {
          tunnel: w329 -> [w337 w352 w363 w376 w389]
          tunnel: [w339 w353 w365 w378 w391] -> w328
          tunnel: w326 -> [w338 w350 w364 w377 w390]
          frame "Open", "Standard", Default {
            w332 = T3."Standard" ("State")
            n143 = property class="VI"(reference=w338, error in=w337) -> (reference out=w335:refnum<vi>, error out=w336:errorcluster, "FP.State"=w334:T3)
            n144 = Not Equal?(x=w334, y=w332) -> (x != y?=w333:bool)
            n145 = case shown="False" w333 {
              tunnel: [w343 w345] -> w339
              tunnel: w336 -> [w342 w345]
              tunnel: w335 -> [w341 _]
              tunnel: w332 -> [w340 _]
              frame True {
                n146 = invoke class="VI" method="FP.Open"(reference=w341, error in=w342, "Activate"=TRUE, "State"=w340) -> (error out=w343:errorcluster)  [unwired: 1 in, 4 out]
              }
              frame False {
              }
            }
          }
          frame "Close", "Closed" {
            n147 = property class="VI"(reference=w350, error in=w352) -> (reference out=w349:refnum<vi>, error out=w351:errorcluster, "FP.State"=w347:T3)
            n148 = Not Equal?(x=w347, y=T3."Closed" ("Front Panel Window:State")) -> (x != y?=w346:bool)
            n149 = case shown="True" w346 {
              tunnel: [w354 w357] -> w353
              tunnel: w351 -> [w354 w356]
              tunnel: w349 -> [_ w355]
              frame False {
              }
              frame True {
                n150 = invoke class="VI" method="FP.Close"(reference=w355, error in=w356) -> (error out=w357:errorcluster)  [unwired: 1 in, 2 out]
              }
            }
          }
          frame "Hidden", "Hide" {
            w358 = T3."Hidden" ("State")
            n151 = property class="VI"(reference=w364, error in=w363) -> (reference out=w361:refnum<vi>, error out=w362:errorcluster, "FP.State"=w360:T3)
            n152 = Not Equal?(x=w360, y=w358) -> (x != y?=w359:bool)
            n153 = case shown="True" w359 {
              tunnel: [w369 w370] -> w365
              tunnel: w362 -> [w368 w370]
              tunnel: w361 -> [w367 _]
              tunnel: w358 -> [w366 _]
              frame True {
                n154 = invoke class="VI" method="FP.Open"(reference=w367, error in=w368, "State"=w366) -> (error out=w369:errorcluster)  [unwired: 2 in, 4 out]
              }
              frame False {
              }
            }
          }
          frame "Minimize", "Minimized" {
            w371 = T3."Minimized" ("State")
            n155 = property class="VI"(reference=w377, error in=w376) -> (reference out=w374:refnum<vi>, error out=w375:errorcluster, "FP.State"=w373:T3)
            n156 = Not Equal?(x=w373, y=w371) -> (x != y?=w372:bool)
            n157 = case shown="True" w372 {
              tunnel: [w382 w383] -> w378
              tunnel: w375 -> [w381 w383]
              tunnel: w374 -> [w380 _]
              tunnel: w371 -> [w379 _]
              frame True {
                n158 = invoke class="VI" method="FP.Open"(reference=w380, error in=w381, "State"=w379) -> (error out=w382:errorcluster)  [unwired: 2 in, 4 out]
              }
              frame False {
              }
            }
          }
          frame "Maximize", "Maximized" {
            w384 = T3."Maximized" ("State")
            n159 = property class="VI"(reference=w390, error in=w389) -> (reference out=w387:refnum<vi>, error out=w388:errorcluster, "FP.State"=w386:T3)
            n160 = Not Equal?(x=w386, y=w384) -> (x != y?=w385:bool)
            n161 = case shown="True" w385 {
              tunnel: [w395 w396] -> w391
              tunnel: w388 -> [w394 w396]
              tunnel: w387 -> [w393 _]
              tunnel: w384 -> [w392 _]
              frame True {
                n162 = invoke class="VI" method="FP.Open"(reference=w393, error in=w394, "State"=w392) -> (error out=w395:errorcluster)  [unwired: 2 in, 4 out]
              }
              frame False {
              }
            }
          }
        }
        n163 = call <vilib>:"Add State(s) to Queue__JKI_lib_State_Machine.vi"("State(s) in (\"\")"=w331) -> ("States Out"=w330:string)  [unwired: 14 in]
      }
      frame "---------- Macro ----------" {
        # "Do not put any code in this frame.\n(It is a separator no-op. You can make a copy of this frame to create a new Macro frame)"
        n164 = call <vilib>:"Add State(s) to Queue__JKI_lib_State_Machine.vi"("State(s) in (\"\")"=w400) -> ("States Out"=w399:string)  [unwired: 14 in]
      }
      frame "Macro: Display Web" {
        n165 = call <vilib>:"Add State(s) to Queue__JKI_lib_State_Machine.vi"("State(s) in Front (\"\")"="Actions: Find Missing Issues\nActions: Update Info\nImages: Check Cache\nActions: Populate Comic Info", "State(s) in (\"\")"=w405) -> ("States Out"=w404:string)  [unwired: 13 in]
      }
      frame "Macro: Update UI" {
        n166 = call <vilib>:"Add State(s) to Queue__JKI_lib_State_Machine.vi"("State(s) in Front (\"\")"="Actions: Populate Series\nActions: Build Series Path\nActions: Populate Current Issues\nActions: Load JSON\nActions: Populate JSON Issues\nMacro: Display Current\nMacro: Display Web\nActions: Check Sync\nActions: Populate New Issues\nActions: Populate Series Info\nMacro: Display New", "State(s) in (\"\")"=w410) -> ("States Out"=w409:string)  [unwired: 13 in]
      }
      frame "Macro: Display Current" {
        n167 = call <vilib>:"Add State(s) to Queue__JKI_lib_State_Machine.vi"("State(s) in Front (\"\")"="Actions: Find Missing Issues\nImages: Clean local Folder\nImages: Expand current\nActions: Update Info\nImages: Display Local Cover", "State(s) in (\"\")"=w415) -> ("States Out"=w414:string)  [unwired: 13 in]
      }
      frame "Macro: Display Moved" {
        n168 = call <vilib>:"Add State(s) to Queue__JKI_lib_State_Machine.vi"("State(s) in Front (\"\")"="Actions: Select Moved", "State(s) in (\"\")"=w420) -> ("States Out"=w419:string)  [unwired: 13 in]
      }
      frame "Macro: Display New" {
        n169 = call <vilib>:"Add State(s) to Queue__JKI_lib_State_Machine.vi"("State(s) in Front (\"\")"="Images: Clean New Folder\nImages: Expand new\nImages: Display New Cover", "State(s) in (\"\")"=w425) -> ("States Out"=w424:string)  [unwired: 13 in]
      }
      frame "Macro: Initialize" {
        w426 = "Data: Initialize\nInitialize Core Data\nUI: Initialize\nUI: Front Panel State >> Open\nData: Init Temp Folders\nMacro: Update UI"  # Data: Initialize Initialize Core Data UI: Initialize UI: Front Panel State >> Open Data: Init Temp Folders Macro: Update UI
        # "Initialization Macro\n(This is called once, when the VI starts)"
        n170 = call <vilib>:"Add State(s) to Queue__JKI_lib_State_Machine.vi"("State(s) in Front (\"\")"=w426, "State(s) in (\"\")"=w430) -> ("States Out"=w429:string)  [unwired: 13 in]
      }
      frame "Macro: Exit" {
        # "Exit Macro\n(This is called once, when the VI exits)"
        n171 = Unbundle By Name(w437) -> ("Core.Close Panel on Exit?"=w436:bool)
        n172 = Select(t="UI: Front Panel State >> Close", s=w436, f="") -> (s? t:f=w433:string)
        n173 = call <vilib>:"Add State(s) to Queue__JKI_lib_State_Machine.vi"("State(s) in (\"\")"=w433, "State(s) at Back (\"\")"="Data: Cleanup\nExit") -> ("States Out"=w431:string)  [unwired: 13 in]
        n174 = call <vilib>:"Add State(s) to Queue__JKI_lib_State_Machine.vi"("State(s) in Front (\"\")"=w431, "State(s) in (\"\")"=w440) -> ("States Out"=w439:string)  [unwired: 13 in]
      }
      frame "---------- Images ----------" {
        n175 = call <vilib>:"Add State(s) to Queue__JKI_lib_State_Machine.vi"("State(s) in (\"\")"=w444) -> ("States Out"=w443:string)  [unwired: 14 in]
      }
      frame "Images: Check Cache" {
        n176 = local read "Marvel Issues"() -> (w463:i32)
        n177 = Unbundle By Name(w449) -> ("comic jsons"=w462:T6[])
        n178 = Index Array(array=w462, index=w463) -> (element=w461:T6)
        n179 = Unbundle By Name(w461) -> ("id"=w459:i32, "images"=w448:cluster{"path":string, "extension":string}[])
        n180 = Array Size(array=w448) -> (size(s)=w447:i32)
        n181 = Format Into String(format string="%d.jpg", w459) -> (resulting string=w458:string)  [unwired: 2 in, 1 out]
        n182 = Greater?(x=w447, y=1) -> (0:w445:bool)
        n183 = Build Path(base path=path "D:/Comics/data/cache", name or relative path=w458) -> (appended path=w452:path)
        n184 = local write "More Avail"(w445) -> ()
        n185 = call <vilib>:"Check if File or Folder Exists.vi"("error in (no error)"=w456, "path"=w452) -> ("error out"=w455:errorcluster, "file or folder exists?"=w454:bool)  [unwired: 7 in, 1 out]
        n186 = case shown="False" w454 {
          tunnel: ["UI: Cursor Set >> Busy\nImages: Download Cover\nUI: Cursor Set >> Idle\nImages: Display Web Cover" "Images: Display Web Cover"] -> w453
          frame False {
          }
          frame True {
          }
        }
        n187 = Bundle By Name(cluster=w449, "display web"=TRUE, "web cover path"=w452) -> (w451:T8)
        n188 = call <vilib>:"Add State(s) to Queue__JKI_lib_State_Machine.vi"("State(s) in Front (\"\")"=w453, "State(s) in (\"\")"=w465) -> ("States Out"=w464:string)  [unwired: 13 in]
      }
      frame "Images: Remove from Cache" {
        n189 = local read "Marvel Issues"() -> (w481:i32)
        n190 = Unbundle By Name(w471) -> ("comic jsons"=w480:T6[])
        n191 = Index Array(array=w480, index=w481) -> (element=w479:T6)
        n192 = Unbundle By Name(w479) -> ("id"=w477:i32)
        n193 = Format Into String(format string="%d.jpg", w477) -> (resulting string=w476:string)  [unwired: 2 in, 1 out]
        n194 = Build Path(base path=path "D:/Comics/data/cache", name or relative path=w476) -> (appended path=w474:path)
        n195 = call <vilib>:"Check if File or Folder Exists.vi"("error in (no error)"=w473, "path"=w474) -> ("error out"=w469:errorcluster, "file or folder exists?"=w472:bool, "dup path"=w470:path)  [unwired: 7 in]
        n196 = case shown="True" w472 {
          tunnel: w470 -> [_ w487]
          tunnel: w469 -> [w484 w486]
          tunnel: [w484 w485] -> w468
          frame False {
          }
          frame True {
            n197 = Delete(path (use dialog)=w487, error in=w486) -> (error out=w485:errorcluster)  [unwired: 3 in, 2 out]
          }
        }
        n198 = call <vilib>:"Add State(s) to Queue__JKI_lib_State_Machine.vi"("State(s) in (\"\")"=w483) -> ("States Out"=w482:string)  [unwired: 14 in]
      }
      frame "Images: Rotate json Image" {
        n199 = local read "Marvel Issues"() -> (w491:i32)
        n200 = Unbundle By Name(w512) -> ("comic jsons"=w490:T6[], "series path"=w494:path)
        n201 = List Folder(path=w494, pattern="comics.*.json", error in=w497) -> (filenames=w496:string[], error out=w492:errorcluster)  [unwired: 1 in, 2 out]
        n202 = in-place {
          n203 = in-place-array #1(w490, w491) -> (w516:T6)
          n204 = in-place {
            n205 = in-place-cluster #2(w516) -> ("images"=w518:cluster{"path":string, "extension":string}[])
            n206 = Rotate 1D Array(1:w518, 2:1 ("n")) -> (0:w517:cluster{"path":string, "extension":string}[])
            n207 = in-place-cluster #2("images"=w517) -> (w515:T6)
          }
          n208 = in-place-array #1(w515) -> (w489:T6[])  [unwired: 1 out]
        }
        n209 = Index Array(array=w496) -> (element=w495:string)  [unwired: 1 in]
        n210 = Build Path(base path=w494, name or relative path=w495) -> (appended path=w493:path)
        n211 = Read from Text File(file (use dialog)=w493, error in=w492) -> (text=w499:string, error out=w502:errorcluster)  [unwired: 2 in, 2 out]
        n212 = Bundle By Name(cluster=w512, "comic jsons"=w489) -> (w511:T8)
        n213 = call "parse.comics_reply.vi"("error in"=w502, "string in"=w499) -> ("error out"=w501:errorcluster, "data"=w500:T10)  [unwired: 8 in]
        n214 = Bundle By Name(cluster=w500, "data.results"=w489) -> (w510:T10)
        n215 = call <vilib>:"Flatten To JSON String.vi"("error in"=w501, "Variant"=w510) -> ("error out"=w509:errorcluster, "JSON String"=w505:string)  [unwired: 8 in]
        n216 = Open/Create/Replace File(file path (use dialog)=w493, error in=w509, operation (0:open)=T5."replace") -> (refnum out=w506:refnum<file>, error out=w507:errorcluster)  [unwired: 3 in, 1 out]
        n217 = Write to Text File(file (use dialog)=w506, text=w505, error in=w507) -> (refnum out=w503:refnum<file>, error out=w504:errorcluster)  [unwired: 1 in, 1 out]
        n218 = Close File(refnum=w503, error in=w504) -> (error out=w488:errorcluster)  [unwired: 1 out]
        n219 = call <vilib>:"Add State(s) to Queue__JKI_lib_State_Machine.vi"("State(s) in (\"\")"=w514) -> ("States Out"=w513:string)  [unwired: 14 in]
      }
      frame "Images: Download Cover" {
        n220 = Unbundle By Name(w523) -> ("json present"=w528:bool, "web cover path"=w529:path, "comic jsons"=w531:T6[])
        n221 = local read "Marvel Issues"() -> (w530:i32)
        n222 = case shown="True" w528 {
          tunnel: w531 -> [_ w556]
          tunnel: w530 -> [_ w555]
          tunnel: w529 -> [_ w545]
          tunnel: w525 -> [w539 w550]
          tunnel: [w539 w549] -> w527
          tunnel: [_ TRUE] -> w526
          tunnel: [_ w541] -> w520
          frame False {
          }
          frame True {
            n223 = Index Array(array=w556, index=w555) -> (element=w554:T6)
            n224 = Unbundle By Name(w554) -> ("images"=w544:cluster{"path":string, "extension":string}[])
            n225 = Index Array(array=w544) -> (element=w553:cluster{"path":string, "extension":string})  [unwired: 1 in]
            n226 = Array Size(array=w544) -> (size(s)=w543:i32)
            n227 = Unbundle By Name(w553) -> ("path"=w552:string, "extension"=w548:string)
            n228 = Greater?(x=w543, y=1) -> (0:w541:bool)
            n229 = Concatenate Strings(w552, "." ("string"), w548) -> (w551:string)
            n230 = call <vilib>:"GET.vi"("output file"=w545, "url"=w551, "error in (no error)"=w550, "timeout (10000)"=2000) -> ("error out"=w549:errorcluster)  [unwired: 8 in, 3 out]
          }
        }
        "More Avail" <- w520
        n231 = case shown="Error 56, 59" w527 {
          selector: w527 -> [w535 w536 w538]
          tunnel: [w535 w536 w537] -> w524
          tunnel: [w534 _ _] -> w521
          tunnel: w526 -> [w534 _ _]
          frame No Error {
          }
          frame Default {
          }
          frame Error {
            n232 = call <vilib>:"Clear Errors.vi"("error in (no error)"=w538) -> ("error out"=w537:errorcluster)  [unwired: 5 in, 1 out]
          }
        }
        n233 = Bundle By Name(cluster=w523, "display web"=w521) -> (w522:T8)
        n234 = call <vilib>:"Add State(s) to Queue__JKI_lib_State_Machine.vi"("State(s) in (\"\")"=w533) -> ("States Out"=w532:string)  [unwired: 14 in]
      }
      frame "Images: Clean New Folder" {
        n235 = Unbundle By Name(w559) -> ("new working folder"=w560:path)
        n236 = call "ClearWorkingDirectory.vi"("error in"=w557, "Working Path"=w560) -> ("error out"=w558:errorcluster)  [unwired: 8 in, 1 out]
        n237 = call <vilib>:"Add State(s) to Queue__JKI_lib_State_Machine.vi"("State(s) in (\"\")"=w562) -> ("States Out"=w561:string)  [unwired: 14 in]
      }
      frame "Images: Clean local Folder" {
        n238 = Unbundle By Name(w565) -> ("local working folder"=w566:path)
        n239 = call "ClearWorkingDirectory.vi"("error in"=w563, "Working Path"=w566) -> ("error out"=w564:errorcluster)  [unwired: 8 in, 1 out]
        n240 = call <vilib>:"Add State(s) to Queue__JKI_lib_State_Machine.vi"("State(s) in (\"\")"=w568) -> ("States Out"=w567:string)  [unwired: 14 in]
      }
      frame "Images: Display Local Cover" {
        n241 = Unbundle By Name(w583) -> ("local working folder"=w590:path)
        n242 = List Folder(path=w590, error in=w582) -> (path out=w588:path, filenames=w589:string[], error out=w587:errorcluster)  [unwired: 2 in, 1 out]
        n243 = Index Array(array=w589) -> (element=w585:string)  [unwired: 1 in]
        n244 = Build Path(base path=w588, name or relative path=w585) -> (appended path=w586:path)
        n245 = call-poly <userlib>:"Strip Path Extension__ogtk.vi"("path"=w585) -> ("extension"=w584:string)  [unwired: 1 out]
        n246 = case shown="\"jpeg\", \"jpg\"" w584 {
          tunnel: w587 -> [w593 w598 w603]
          tunnel: [_ w597 w602] -> w581
          tunnel: [_ w596 w601] -> w574
          tunnel: [w593 w595 w600] -> w572
          tunnel: w586 -> [_ w594 w599]
          frame Default {
          }
          frame "jpeg", "jpg" {
            n247 = call <vilib>:"Read JPEG File.vi"("error in (no error)"=w598, "path to JPEG file"=w594) -> ("error out"=w595:errorcluster, "image data"=w596:T11)  [unwired: 7 in, 1 out]
            n248 = call <vilib>:"Draw Flattened Pixmap.vi"("image data"=w596) -> ("new picture"=w597:picture)  [unwired: 8 in]
          }
          frame "png" {
            n249 = call <vilib>:"Read PNG File.vi"("error in (no error)"=w603, "path to PNG file"=w599) -> ("error out"=w600:errorcluster, "image data"=w601:T11)  [unwired: 7 in, 1 out]
            n250 = call <vilib>:"Draw Flattened Pixmap.vi"("image data"=w601) -> ("new picture"=w602:picture)  [unwired: 8 in]
          }
        }
        "current issue cover" <- w581
        n251 = property on="current issue cover" class="Pict"(error in=w572) -> (error out=w571:errorcluster, "Draw Area Size"=w573:T12)  [unwired: 1 in, 1 out]
        n252 = Unbundle By Name(w574) -> ("Rectangle.right"=w578:i16, "Rectangle.bottom"=w577:i16)
        n253 = Unbundle By Name(w573) -> ("Width"=w580:u32, "Height"=w579:u32)
        n254 = Divide(x=w580, y=w578) -> (x/y=w576:dbl)
        n255 = Divide(x=w579, y=w577) -> (x/y=w575:dbl)
        n256 = Max & Min(x=w576, y=w575) -> (min(x,y)=w570:dbl)  [unwired: 1 out]
        n257 = property on="current issue cover" class="Pict"(error in=w571, "ZoomFactor"=w570) -> (error out=w569:errorcluster)  [unwired: 1 in, 1 out]
        n258 = call <vilib>:"Add State(s) to Queue__JKI_lib_State_Machine.vi"("State(s) in (\"\")"=w592) -> ("States Out"=w591:string)  [unwired: 14 in]
      }
      frame "Images: Display New Cover" {
        n259 = Unbundle By Name(w618) -> ("new working folder"=w625:path)
        n260 = List Folder(path=w625, error in=w617) -> (path out=w623:path, filenames=w624:string[], error out=w622:errorcluster)  [unwired: 2 in, 1 out]
        n261 = Index Array(array=w624) -> (element=w620:string)  [unwired: 1 in]
        n262 = Build Path(base path=w623, name or relative path=w620) -> (appended path=w621:path)
        n263 = call-poly <userlib>:"Strip Path Extension__ogtk.vi"("path"=w620) -> ("extension"=w619:string)  [unwired: 1 out]
        n264 = case shown="\"jpeg\", \"jpg\"" w619 {
          tunnel: w622 -> [w628 w633 w638]
          tunnel: [_ w632 w637] -> w604
          tunnel: [_ w631 w636] -> w610
          tunnel: [w628 w630 w635] -> w608
          tunnel: w621 -> [_ w629 w634]
          frame Default {
          }
          frame "jpeg", "jpg" {
            n265 = call <vilib>:"Read JPEG File.vi"("error in (no error)"=w633, "path to JPEG file"=w629) -> ("error out"=w630:errorcluster, "image data"=w631:T11)  [unwired: 7 in, 1 out]
            n266 = call <vilib>:"Draw Flattened Pixmap.vi"("image data"=w631) -> ("new picture"=w632:picture)  [unwired: 8 in]
          }
          frame "png" {
            n267 = call <vilib>:"Read PNG File.vi"("error in (no error)"=w638, "path to PNG file"=w634) -> ("error out"=w635:errorcluster, "image data"=w636:T11)  [unwired: 7 in, 1 out]
            n268 = call <vilib>:"Draw Flattened Pixmap.vi"("image data"=w636) -> ("new picture"=w637:picture)  [unwired: 8 in]
          }
        }
        "new issue cover" <- w604
        n269 = property on="new issue cover" class="Pict"(error in=w608) -> (error out=w607:errorcluster, "Draw Area Size"=w609:T12)  [unwired: 1 in, 1 out]
        n270 = Unbundle By Name(w610) -> ("Rectangle.right"=w614:i16, "Rectangle.bottom"=w613:i16)
        n271 = Unbundle By Name(w609) -> ("Width"=w616:u32, "Height"=w615:u32)
        n272 = Divide(x=w616, y=w614) -> (x/y=w612:dbl)
        n273 = Divide(x=w615, y=w613) -> (x/y=w611:dbl)
        n274 = Max & Min(x=w612, y=w611) -> (min(x,y)=w606:dbl)  [unwired: 1 out]
        n275 = property on="new issue cover" class="Pict"(error in=w607, "ZoomFactor"=w606) -> (error out=w605:errorcluster)  [unwired: 1 in, 1 out]
        n276 = call <vilib>:"Add State(s) to Queue__JKI_lib_State_Machine.vi"("State(s) in (\"\")"=w627) -> ("States Out"=w626:string)  [unwired: 14 in]
      }
      frame "Images: Display Web Cover" {
        n277 = Unbundle By Name(w645) -> ("web cover path"=w648:path, "json present"=w646:bool, "display web"=w640:bool)
        n278 = And(x=w646, y=w640) -> (x .and. y?=w647:bool)
        n279 = case shown="True" w647 {
          tunnel: [_ w674] -> w643
          tunnel: [w669 w673] -> w641
          tunnel: [_ w672] -> w642
          tunnel: w644 -> [w669 w671]
          tunnel: w648 -> [_ w670]
          frame False {
          }
          frame True {
            n280 = call <vilib>:"Read JPEG File.vi"("error in (no error)"=w671, "path to JPEG file"=w670) -> ("error out"=w673:errorcluster, "image data"=w674:T11)  [unwired: 7 in, 1 out]
            n281 = call <vilib>:"Draw Flattened Pixmap.vi"("image data"=w674) -> ("new picture"=w672:picture)  [unwired: 8 in]
          }
        }
        "json issue cover" <- w642
        n282 = case shown="No Error" w641 {
          selector: w641 -> [w653 w665 w668]
          tunnel: [w655 w665 w667] -> w649
          tunnel: w643 -> [w654 _ _]
          tunnel: w640 -> [w652 _ _]
          tunnel: [w652 _ _] -> w639
          frame No Error {
            n283 = property on="json issue cover" class="Pict"(error in=w653) -> (error out=w657:errorcluster, "Draw Area Size"=w658:T12)  [unwired: 1 in, 1 out]
            n284 = Unbundle By Name(w654) -> ("Rectangle.right"=w662:i16, "Rectangle.bottom"=w661:i16)
            n285 = Unbundle By Name(w658) -> ("Width"=w664:u32, "Height"=w663:u32)
            n286 = Divide(x=w664, y=w662) -> (x/y=w660:dbl)
            n287 = Divide(x=w663, y=w661) -> (x/y=w659:dbl)
            n288 = Max & Min(x=w660, y=w659) -> (min(x,y)=w656:dbl)  [unwired: 1 out]
            n289 = property on="json issue cover" class="Pict"(error in=w657, "ZoomFactor"=w656) -> (error out=w655:errorcluster)  [unwired: 1 in, 1 out]
          }
          frame Default {
          }
          frame Error {
            n290 = call <vilib>:"Clear Errors.vi"("error in (no error)"=w668, "specific error code to clear (0: all)"=7) -> ("error out"=w667:errorcluster)  [unwired: 4 in, 1 out]
          }
        }
        "Available?" <- w639
        n291 = call <vilib>:"Add State(s) to Queue__JKI_lib_State_Machine.vi"("State(s) in (\"\")"=w651) -> ("States Out"=w650:string)  [unwired: 14 in]
      }
      frame "Images: Expand current" {
        n292 = Unbundle By Name(w682) -> ("series path"=w687:path, "local working folder"=w689:path)
        n293 = property on="Collected Issues" class="LstBox (strict)"(error in=w683) -> (error out=w679:errorcluster, "Item Names"=w686:string[], "Value"=w685:i32)  [unwired: 1 in, 1 out]
        n294 = Index Array(array=w686, index=w685) -> (element=w688:string)
        n295 = Build Path(base path=w687, name or relative path=w688) -> (appended path=w678:path)
        n296 = call <vilib>:"Check if File or Folder Exists.vi"("error in (no error)"=w679, "path"=w678) -> ("error out"=w676:errorcluster, "file or folder exists?"=w675:bool, "dup path"=w677:path)  [unwired: 7 in]
        n297 = case shown="True" w675 {
          tunnel: w689 -> [_ w702]
          tunnel: [w692 w701] -> w684
          tunnel: [_ w697] -> w681
          tunnel: w678 -> [_ w696]
          tunnel: w677 -> [_ w695]
          tunnel: w676 -> [w692 w694]
          frame False {
          }
          frame True {
            n298 = File/Directory Info(path=w695, error in=w694) -> (size=w699:i64, error out=w700:errorcluster)  [unwired: 5 out]
            n299 = call "PathToQuotedString.vi"("Path"=w696) -> ("String"=w704:string)  [unwired: 10 in]
            n300 = call "PathToQuotedString.vi"("Path"=w702) -> ("String"=w705:string)  [unwired: 10 in]
            n301 = Format Into String(format string="%.3p", w699) -> (resulting string=w697:string)  [unwired: 2 in, 1 out]
            n302 = Format Into String(format string="%s e %s -o%s -r", error in=w700, "\"C:\\Program Files\\7-Zip\\7z.exe\"" ("input 1"), w704, w705) -> (resulting string=w706:string, error out=w707:errorcluster)  [unwired: 1 in]
            n303 = call <vilib>:"System Exec.vi"("run minimized? (F)"=TRUE, "error in (no error)"=w707, "command line"=w706) -> ("error out"=w701:errorcluster)  [unwired: 5 in, 3 out]
          }
        }
        n304 = Bundle By Name(cluster=w682, "current size"=w681) -> (w680:T8)
        n305 = call <vilib>:"Add State(s) to Queue__JKI_lib_State_Machine.vi"("State(s) in (\"\")"=w691) -> ("States Out"=w690:string)  [unwired: 14 in]
      }
      frame "Images: Expand new" {
        n306 = property on="New Issues" class="LstBox (strict)"(error in=w710) -> (error out=w713:errorcluster, "Item Names"=w715:string[], "Value"=w714:i32)  [unwired: 1 in, 1 out]
        n307 = Unbundle By Name(w712) -> ("new working folder"=w718:path)
        n308 = local read "New Comics"() -> (w709:path)
        n309 = Index Array(array=w715, index=w714) -> (element=w717:string)
        n310 = Build Path(base path=w709, name or relative path=w717) -> (appended path=w716:path)
        n311 = call "PathToQuotedString.vi"("Path"=w718) -> ("String"=w721:string)  [unwired: 10 in]
        n312 = call "PathToQuotedString.vi"("Path"=w716) -> ("String"=w720:string)  [unwired: 10 in]
        n313 = Format Into String(format string="%s e %s -o%s -r", error in=w713, "\"C:\\Program Files\\7-Zip\\7z.exe\"" ("input 1"), w720, w721) -> (resulting string=w723:string, error out=w724:errorcluster)  [unwired: 1 in]
        n314 = call <vilib>:"System Exec.vi"("run minimized? (F)"=TRUE, "error in (no error)"=w724, "command line"=w723) -> ("error out"=w711:errorcluster)  [unwired: 5 in, 3 out]
        n315 = call <vilib>:"Add State(s) to Queue__JKI_lib_State_Machine.vi"("State(s) in (\"\")"=w727) -> ("States Out"=w726:string)  [unwired: 14 in]
      }
      frame "---------- Actions ----------" {
        n316 = call <vilib>:"Add State(s) to Queue__JKI_lib_State_Machine.vi"("State(s) in (\"\")"=w731) -> ("States Out"=w730:string)  [unwired: 14 in]
      }
      frame "Actions: Populate Comic Info" {
        n317 = Unbundle By Name(w744) -> ("comic jsons"=w743:T6[])
        n318 = property on="Marvel Issues" class="LstBox (strict)"(error in=w741) -> ("Value"=w742:i32)  [unwired: 1 in, 2 out]
        n319 = Index Array(array=w743, index=w742) -> (element=w740:T6)
        n320 = Unbundle By Name(w740) -> ("title"=w746:string, "description"=w745:string, "dates"=w738:cluster{"type":string, "date":string}[], "creators.items"=w733:T13, "characters.items"=w734:cluster{"resourceURI":string, "name":string}[])
        n321 = call "parse.onsaleDate.vi"("dates"=w738) -> ("date string"=w737:string)  [unwired: 1 out]
        n322 = for {
          tunnel: w733 -> [w750] mode=indexing
          tunnel: [w749] -> w732 mode=indexing
          n323 = Unbundle By Name(w750) -> ("name"=w749:string)
        }
        n324 = for {
          tunnel: w734 -> [w752] mode=indexing
          tunnel: [w751] -> w735 mode=indexing
          n325 = Unbundle By Name(w752) -> ("name"=w751:string)
        }
        n326 = Bundle By Name(cluster=T1 {"rel date"="", "title"="", "description"="", "creators"=[""], "characters"=[""]} ("comic info"), "title"=w746, "description"=w745, "rel date"=w737, "creators"=w732, "characters"=w735) -> (w736:T1)
        n327 = local write "comic info"(w736) -> ()
        n328 = call <vilib>:"Add State(s) to Queue__JKI_lib_State_Machine.vi"("State(s) in (\"\")"=w748) -> ("States Out"=w747:string)  [unwired: 14 in]
      }
      frame "Actions: Populate Series Info" {
        n329 = Unbundle By Name(w762) -> ("series json.id"=w759:i32, "series json.title"=w758:string, "series json.description"=w757:string, "series json.startYear"=w756:i32, "series json.endYear"=w755:i32, "series json.type"=w754:string, "series json.tags"=w753:string[])
        n330 = Bundle By Name(cluster=T2 {"seriesType"="", "title"="", "id"=0, "description"="", "start year"=0, "end year"=0, "tags"=[]} ("series info"), "id"=w759, "title"=w758, "description"=w757, "start year"=w756, "end year"=w755, "seriesType"=w754, "tags"=w753) -> (w760:T2)
        n331 = local write "series info"(w760) -> ()
        n332 = call <vilib>:"Add State(s) to Queue__JKI_lib_State_Machine.vi"("State(s) in (\"\")"=w765) -> ("States Out"=w764:string)  [unwired: 14 in]
      }
      frame "Actions: Apply Series Changes" {
        n333 = local read "series info"() -> (w790:T2)
        n334 = Unbundle By Name(w782) -> ("series path"=w775:path, "series json"=w789:T7)
        n335 = Unbundle By Name(w790) -> ("id"=w777:u32, "title"=w788:string, "description"=w787:string, "start year"=w786:u32, "end year"=w785:u32, "seriesType"=w784:string, "tags"=w783:string[])
        n336 = Format Into String(format string="series.%d.json", w777) -> (resulting string=w776:string)  [unwired: 2 in, 1 out]
        n337 = Bundle By Name(cluster=w789, "id"=w777, "title"=w788, "description"=w787, "startYear"=w786, "endYear"=w785, "type"=w784, "tags"=w783) -> (w780:T7)
        n338 = Build Path(base path=w775, name or relative path=w776) -> (appended path=w774:path)
        n339 = Bundle By Name(cluster=w782, "series json"=w780) -> (w781:T8)
        n340 = call <vilib>:"Flatten To JSON String.vi"("error in"=w779, "Variant"=w780) -> ("error out"=w769:errorcluster, "JSON String"=w772:string)  [unwired: 8 in]
        n341 = Open/Create/Replace File(file path (use dialog)=w774, error in=w769, operation (0:open)=T5."replace or create") -> (refnum out=w771:refnum<file>, error out=w770:errorcluster)  [unwired: 3 in, 1 out]
        n342 = Write to Text File(file (use dialog)=w771, text=w772, error in=w770) -> (refnum out=w767:refnum<file>, error out=w768:errorcluster)  [unwired: 1 in, 1 out]
        n343 = Close File(refnum=w767, error in=w768) -> (error out=w766:errorcluster)  [unwired: 1 out]
        n344 = call <vilib>:"Add State(s) to Queue__JKI_lib_State_Machine.vi"("State(s) in (\"\")"=w792) -> ("States Out"=w791:string)  [unwired: 14 in]
      }
      frame "Actions: Rename File" {
        n345 = Unbundle By Name(w797) -> ("series path"=w796:path, "json present"=w793:bool)
        n346 = case shown="True" w793 {
          tunnel: w796 -> [_ w806]
          tunnel: w795 -> [w800 w802]
          tunnel: [w800 w801] -> w794
          frame False {
          }
          frame True {
            n347 = property on="Collected Issues" class="LstBox (strict)"(error in=w802) -> (error out=w805:errorcluster, "Item Names"=w814:string[], "Value"=w813:i32)  [unwired: 1 in, 1 out]
            n348 = property on="Marvel Issues" class="LstBox (strict)"(error in=w802) -> (error out=w803:errorcluster, "Item Names"=w809:string[], "Value"=w808:i32)  [unwired: 1 in, 1 out]
            n349 = Merge Errors(w805, w803) -> (w804:errorcluster)
            n350 = Index Array(array=w814, index=w813) -> (element=w810:string)
            n351 = Index Array(array=w809, index=w808) -> (element=w807:string)
            n352 = Build Path(base path=w806, name or relative path=w810) -> (appended path=w812:path)
            n353 = Build Path(base path=w806, name or relative path=w807) -> (appended path=w811:path)
            n354 = Move(source path=w812, error in=w804, 10:w811) -> (error out=w801:errorcluster)  [unwired: 2 in, 2 out]
          }
        }
        n355 = call <vilib>:"Add State(s) to Queue__JKI_lib_State_Machine.vi"("State(s) in (\"\")"=w799) -> ("States Out"=w798:string)  [unwired: 14 in]
      }
      frame "Actions: Rename All" {
        n356 = Unbundle By Name(w819) -> ("series path"=w818:path, "json present"=w815:bool)
        n357 = case shown="True" w815 {
          tunnel: w818 -> [_ w824]
          tunnel: w817 -> [w822 w828]
          tunnel: [w822 w823] -> w816
          frame False {
          }
          frame True {
            n358 = property on="Collected Issues" class="LstBox (strict)"(error in=w828) -> (error out=w830:errorcluster, "Item Names"=w825:string[])  [unwired: 1 in, 1 out]
            n359 = property on="Marvel Issues" class="LstBox (strict)"(error in=w828) -> (error out=w829:errorcluster, "Item Names"=w826:string[])  [unwired: 1 in, 1 out]
            n360 = Merge Errors(w830, w829) -> (w827:errorcluster)
            n361 = for {
              tunnel: w826 -> [w831] mode=indexing
              tunnel: w825 -> [w835] mode=indexing
              tunnel: w824 -> [w837]
              shift-right: [w836] -> w823
              shift-left: w827 -> [w838]
              n362 = Build Path(base path=w837, name or relative path=w835) -> (appended path=w834:path)
              n363 = Build Path(base path=w837, name or relative path=w831) -> (appended path=w833:path)
              n364 = Not Equal?(x=w833, y=w834) -> (x != y?=w832:bool)
              n365 = case shown="True" w832 {
                tunnel: w838 -> [w839 w843]
                tunnel: [w839 w842] -> w836
                tunnel: w834 -> [_ w841]
                tunnel: w833 -> [_ w840]
                frame False {
                }
                frame True {
                  n366 = Move(source path=w841, error in=w843, 10:w840) -> (error out=w842:errorcluster)  [unwired: 2 in, 2 out]
                }
              }
            }
          }
        }
        n367 = call <vilib>:"Add State(s) to Queue__JKI_lib_State_Machine.vi"("State(s) in (\"\")"=w821) -> ("States Out"=w820:string)  [unwired: 14 in]
      }
      frame "Actions: Scan for New" {
        n368 = call "GetAllComicsBySeries.vi"("Run as sub"=TRUE, "error in (no error)"=w845) -> ("error IO"=w846:errorcluster)  [unwired: 9 in]
        n369 = call <vilib>:"Add State(s) to Queue__JKI_lib_State_Machine.vi"("State(s) in (\"\")"=w849) -> ("States Out"=w848:string)  [unwired: 14 in]
      }
      frame "Actions: Delete json Issue" {
        n370 = call "Display Message to User"("error in (no error)"=w852) -> ("error out"=w854:errorcluster, "OK"=w853:bool)  [unwired: 9 in]
        n371 = case shown="True" w853 {
          tunnel: w855 -> [w858 w860]
          tunnel: w854 -> [w859 w863]
          tunnel: [w859 w862] -> w851
          tunnel: [w858 w861] -> w850
          frame False {
          }
          frame True {
            n372 = Unbundle By Name(w860) -> ("comic jsons"=w867:T6[], "series path"=w869:path)
            n373 = local read "Marvel Issues"() -> (w868:i32)
            n374 = call <vilib>:"Recursive File List.vi"("pattern"="comics.*.json", "error in (no error)"=w863, "Folder Path"=w869) -> ("error out"=w871:errorcluster, "All Files in Dir"=w870:path[])  [unwired: 4 in, 3 out]
            n375 = Index Array(array=w870) -> (element=w875:path)  [unwired: 1 in]
            n376 = Delete From Array(array=w867, length=1, index=w868) -> (array with subset deleted=w872:T6[])  [unwired: 1 out]
            n377 = Read from Text File(file (use dialog)=w875, error in=w871) -> (text=w884:string, error out=w881:errorcluster)  [unwired: 2 in, 2 out]
            n378 = Bundle By Name(cluster=w860, "comic jsons"=w872) -> (w861:T8)
            n379 = call "parse.comics_reply.vi"("error in"=w881, "string in"=w884) -> ("error out"=w882:errorcluster, "data"=w883:T10)  [unwired: 8 in]
            n380 = Bundle By Name(cluster=w883, "data.results"=w872) -> (w873:T10)
            n381 = call <vilib>:"Flatten To JSON String.vi"("error in"=w882, "Variant"=w873) -> ("error out"=w874:errorcluster, "JSON String"=w878:string)  [unwired: 8 in]
            n382 = Open/Create/Replace File(file path (use dialog)=w875, error in=w874, operation (0:open)=T5."replace") -> (refnum out=w877:refnum<file>, error out=w876:errorcluster)  [unwired: 3 in, 1 out]
            n383 = Write to Text File(file (use dialog)=w877, text=w878, error in=w876) -> (refnum out=w880:refnum<file>, error out=w879:errorcluster)  [unwired: 1 in, 1 out]
            n384 = Close File(refnum=w880, error in=w879) -> (error out=w862:errorcluster)  [unwired: 1 out]
          }
        }
        n385 = call <vilib>:"Add State(s) to Queue__JKI_lib_State_Machine.vi"("State(s) in (\"\")"=w857) -> ("States Out"=w856:string)  [unwired: 14 in]
      }
      frame "Actions: Rename json Title" {
        n386 = property on="Marvel Issues" class="LstBox (strict)"() -> ("Item Names"=w887:string[], "Value"=w886:i32)  [unwired: 2 in, 2 out]
        n387 = Index Array(array=w887, index=w886) -> (element=w885:string)
        n388 = call "dialog.change.string.vi"("Issue Name"=w885) -> ("apply?"=w890:bool, "issue name out"=w888:string)  [unwired: 9 in]
        n389 = case shown="True" w890 {
          tunnel: w893 -> [w896 w898]
          tunnel: [w896 w922] -> w891
          tunnel: [w897 w908] -> w892
          tunnel: w889 -> [w897 w903]
          tunnel: w888 -> [_ w899]
          frame False {
          }
          frame True {
            n390 = Unbundle By Name(w898) -> ("comic jsons"=w902:T6[], "series path"=w921:path)
            n391 = local read "Marvel Issues"() -> (w900:i32)
            n392 = call <vilib>:"Recursive File List.vi"("pattern"="comics.*.json", "error in (no error)"=w903, "Folder Path"=w921) -> ("error out"=w918:errorcluster, "All Files in Dir"=w919:path[])  [unwired: 4 in, 3 out]
            n393 = call "rename.single.title.vi"("index"=w900, "title"=w899, "comic jsons"=w902) -> ("comic jsons 2"=w901:T6[])  [unwired: 8 in]
            n394 = Index Array(array=w919) -> (element=w915:path)  [unwired: 1 in]
            n395 = Read from Text File(file (use dialog)=w915, error in=w918) -> (text=w904:string, error out=w907:errorcluster)  [unwired: 2 in, 2 out]
            n396 = Bundle By Name(cluster=w898, "comic jsons"=w901) -> (w922:T8)
            n397 = call "parse.comics_reply.vi"("error in"=w907, "string in"=w904) -> ("error out"=w906:errorcluster, "data"=w905:T10)  [unwired: 8 in]
            n398 = Bundle By Name(cluster=w905, "data.results"=w901) -> (w917:T10)
            n399 = call <vilib>:"Flatten To JSON String.vi"("error in"=w906, "Variant"=w917) -> ("error out"=w916:errorcluster, "JSON String"=w911:string)  [unwired: 8 in]
            n400 = Open/Create/Replace File(file path (use dialog)=w915, error in=w916, operation (0:open)=T5."replace") -> (refnum out=w912:refnum<file>, error out=w913:errorcluster)  [unwired: 3 in, 1 out]
            n401 = Write to Text File(file (use dialog)=w912, text=w911, error in=w913) -> (refnum out=w909:refnum<file>, error out=w910:errorcluster)  [unwired: 1 in, 1 out]
            n402 = Close File(refnum=w909, error in=w910) -> (error out=w908:errorcluster)  [unwired: 1 out]
          }
        }
        n403 = call <vilib>:"Add State(s) to Queue__JKI_lib_State_Machine.vi"("State(s) in (\"\")"=w895) -> ("States Out"=w894:string)  [unwired: 14 in]
      }
      frame "Actions: Check Sync" {
        n404 = Unbundle By Name(w928) -> ("json present"=w927:bool)
        n405 = case shown="True" w927 {
          tunnel: w926 -> [w931 w943]
          tunnel: [w931 w941] -> w925
          tunnel: [_ w939] -> w924
          tunnel: [_ w932] -> w923
          frame False {
          }
          frame True {
            n406 = property on="Collected Issues" class="LstBox (strict)"(error in=w943) -> (error out=w942:errorcluster, "Item Names"=w940:string[])  [unwired: 1 in, 1 out]
            n407 = property on="New Issues" class="LstBox (strict)"() -> ("Item Names"=w935:string[])  [unwired: 2 in, 2 out]
            n408 = property on="Marvel Issues" class="LstBox (strict)"(error in=w942) -> (error out=w941:errorcluster, "Item Names"=w938:string[])  [unwired: 1 in, 1 out]
            n409 = Empty Array?(array=w935) -> (empty?=w933:bool)
            n410 = Equal?(x=w940, y=w938) -> (x = y?=w939:bool)
            n411 = Array Size(array=w935) -> (size(s)=w937:i32)
            n412 = Array Size(array=w938) -> (size(s)=w936:i32)
            n413 = Equal?(x=w937, y=w936) -> (x = y?=w934:bool)
            n414 = Or(x=w933, y=w934) -> (x .or. y?=w932:bool)
          }
        }
        "synced" <- w924
        "matching count" <- w923
        n415 = call <vilib>:"Add State(s) to Queue__JKI_lib_State_Machine.vi"("State(s) in (\"\")"=w930) -> ("States Out"=w929:string)  [unwired: 14 in]
      }
      frame "Actions: Create New Folder" {
        n416 = call-poly <userlib>:"Strip Path Extension__ogtk.vi"("path"="json file path") -> ("extension"=w953:string)  [unwired: 1 out]
        n417 = call <vilib>:"Check if File or Folder Exists.vi"("error in (no error)"=w945, "path"="json file path") -> ("error out"=w950:errorcluster, "file or folder exists?"=w948:bool, "dup path"=w951:path)  [unwired: 7 in]
        n418 = Equal?(x="json", y=w953) -> (x = y?=w949:bool)
        n419 = And(x=w949, y=w948) -> (x .and. y?=w947:bool)
        n420 = case shown="True" w947 {
          tunnel: [w957 w960] -> w944
          tunnel: w951 -> [_ w959]
          tunnel: w950 -> [w957 w958]
          frame False {
          }
          frame True {
            n421 = call "CreateFolderFromJSON.vi"("error in"=w958, "json file path"=w959) -> ("error out"=w960:errorcluster)  [unwired: 9 in]
          }
        }
        n422 = call <vilib>:"Add State(s) to Queue__JKI_lib_State_Machine.vi"("State(s) in (\"\")"=w956) -> ("States Out"=w955:string)  [unwired: 14 in]
      }
      frame "Actions: Find Missing Issues" {
        n423 = property on="Collected Issues" class="LstBox (strict)"(error in=w964) -> (error out=w963:errorcluster, "Item Names"=w977:string[])  [unwired: 1 in, 1 out]
        n424 = property on="Marvel Issues" class="LstBox (strict)"(error in=w964) -> (error out=w962:errorcluster, "Item Names"=w976:string[])  [unwired: 1 in, 1 out]
        n425 = for {
          tunnel: w977 -> [w994] mode=indexing
          tunnel: [w993] -> w975 mode=indexing
          n426 = call "ParseIssueNumber.vi"("String"=w994) -> ("Numeric"=w993:dbl)
        }
        n427 = for {
          tunnel: w976 -> [w988] mode=indexing
          tunnel: [w987] -> w970 mode=indexing
          n428 = call "ParseIssueNumber.vi"("String"=w988) -> ("Numeric"=w987:dbl)
        }
        n429 = Merge Errors(w963, w962) -> (w961:errorcluster)
        n430 = for {
          tunnel: w970 -> [w991] mode=indexing
          tunnel: w975 -> [w992]
          tunnel: [w991] -> w974 mode=indexing if=w989
          n431 = Search 1D Array(1D array=w992, element=w991) -> (index of element=w990:i32)  [unwired: 1 in]
          n432 = Less Than 0?(x=w990) -> (x < 0?=w989:bool)
        }
        n433 = for {
          tunnel: w975 -> [w985] mode=indexing
          tunnel: w970 -> [w986]
          tunnel: [w985] -> w973 mode=indexing if=w983
          n434 = Search 1D Array(1D array=w986, element=w985) -> (index of element=w984:i32)  [unwired: 1 in]
          n435 = Less Than 0?(x=w984) -> (x < 0?=w983:bool)
        }
        n436 = call-poly <userlib>:"Remove Duplicates from 1D Array__ogtk.vi"("Input Array"=w970) -> ("indices of removed elements"=w972:i32[])  [unwired: 1 out]
        n437 = for {
          tunnel: w970 -> [w982]
          tunnel: w972 -> [w981] mode=indexing
          tunnel: [w980] -> w971 mode=indexing
          n438 = Index Array(array=w982, index=w981) -> (element=w980:dbl)
        }
        n439 = call "SeriesStringGenerator.vi"("Array"=w974) -> ("series string"=w968:string)
        n440 = call "SeriesStringGenerator.vi"("Array"=w973) -> ("series string"=w967:string)
        n441 = call "SeriesStringGenerator.vi"("Array"=w971) -> ("series string"=w966:string)
        n442 = Bundle By Name(cluster=w969, "current missing"=w968, "json missing"=w967, "json dup"=w966) -> (w965:T8)
        n443 = call <vilib>:"Add State(s) to Queue__JKI_lib_State_Machine.vi"("State(s) in (\"\")"=w979) -> ("States Out"=w978:string)  [unwired: 14 in]
      }
      frame "Actions: Update Info" {
        n444 = Unbundle By Name(w1012) -> ("current size"=w1000:string, "current missing"=w1008:string, "json missing"=w1009:string, "json dup"=w1010:string, "json present"=w1011:bool, "comic jsons"=w1014:T6[])
        n445 = local read "Marvel Issues"() -> (w1013:i32)
        n446 = case shown="True" w1011 {
          tunnel: w1014 -> [_ w1029]
          tunnel: w1013 -> [_ w1028]
          tunnel: w1010 -> [w1020 w1023]
          tunnel: w1009 -> [w1019 w1022]
          tunnel: [w1017 w1021] -> w1003
          frame False {
            w1018 = ""
            n447 = Build Array(w1018, w1018, w1019, w1020) -> (w1017:string[])
          }
          frame True {
            n448 = Index Array(array=w1029, index=w1028) -> (element=w1027:T6)
            n449 = Unbundle By Name(w1027) -> ("dates"=w1026:cluster{"type":string, "date":string}[], "upc"=w1024:string)
            n450 = call "parse.onsaleDate.vi"("dates"=w1026) -> ("date string"=w1025:string)  [unwired: 1 out]
            n451 = Build Array(w1025, w1024, w1022, w1023) -> (w1021:string[])
          }
        }
        n452 = Build Array(w1008) -> (w998:string[])
        n453 = Build Array(w1000) -> (w996:string[])
        n454 = Build Array(w998, w996) -> (w997:string[][])
        n455 = property on="current details" class="MCListbox (strict)"(error in=w995, "ItemNames"=w997, "Value"=-1 ("current details")) -> (error out=w1007:errorcluster)  [unwired: 1 in, 1 out]
        n456 = Build Array(w1003) -> (w1002:string[][])
        n457 = Transpose 2D Array(2D array=w1002) -> (transposed array=w1001:string[][])
        n458 = property on="json details" class="MCListbox (strict)"(error in=w995, "ItemNames"=w1001, "Value"=-1 ("comic info")) -> (error out=w1004:errorcluster)  [unwired: 1 in, 1 out]
        n459 = Merge Errors(w1007, w1004) -> (w1006:errorcluster)
        n460 = call <vilib>:"Add State(s) to Queue__JKI_lib_State_Machine.vi"("State(s) in (\"\")"=w1016) -> ("States Out"=w1015:string)  [unwired: 14 in]
      }
      frame "Actions: Select Moved" {
        n461 = disable-structure shown="Enabled" {
          disable-tunnel: [w1036 w1041] -> w1031
          disable-tunnel: w1030 -> [w1035 w1041]
          frame Disabled {
            n462 = property on="Collected Issues" class="LstBox (strict)"(error in=w1035) -> (error out=w1037:errorcluster, "Item Names"=w1040:string[])  [unwired: 1 in, 1 out]
            n463 = Array Size(array=w1040) -> (size(s)=w1039:i32)
            n464 = Decrement(x=w1039) -> (x-1=w1038:i32)
            n465 = property on="Collected Issues" class="LstBox (strict)"(error in=w1037, "Val(Sgnl)"=w1038) -> (error out=w1036:errorcluster)  [unwired: 1 in, 1 out]
          }
          frame Enabled {
          }
        }
        n466 = call <vilib>:"Add State(s) to Queue__JKI_lib_State_Machine.vi"("State(s) in (\"\")"=w1034) -> ("States Out"=w1033:string)  [unwired: 14 in]
      }
      frame "Actions: Move Selected" {
        n467 = Unbundle By Name(w1056) -> ("series path"=w1054:path)
        n468 = property on="New Issues" class="LstBox (strict)"(error in=w1050) -> (error out=w1053:errorcluster, "Item Names"=w1062:string[], "Value"=w1061:i32)  [unwired: 1 in, 1 out]
        n469 = property on="Marvel Issues" class="LstBox (strict)"(error in=w1050) -> (error out=w1052:errorcluster, "Item Names"=w1057:string[], "Value"=w1058:i32)  [unwired: 1 in, 1 out]
        n470 = local read "New Comics"() -> (w1060:path)
        n471 = Index Array(array=w1062, index=w1061) -> (element=w1059:string)
        n472 = Index Array(array=w1057, index=w1058) -> (element=w1055:string)
        n473 = Build Path(base path=w1060, name or relative path=w1059) -> (appended path=w1051:path)
        n474 = Build Path(base path=w1054, name or relative path=w1055) -> (appended path=w1044:path)
        n475 = Merge Errors(w1053, w1052) -> (w1048:errorcluster)
        n476 = call <vilib>:"Check if File or Folder Exists.vi"("error in (no error)"=w1048, "path"=w1044) -> ("error out"=w1046:errorcluster, "file or folder exists?"=w1047:bool, "dup path"=w1045:path)  [unwired: 7 in]
        n477 = case shown="False" w1047 {
          tunnel: w1046 -> [w1065 w1070]
          tunnel: w1045 -> [w1066 w1069]
          tunnel: [w1066 w1068] -> w1043
          tunnel: [w1065 w1067] -> w1042
          frame False {
          }
          frame True {
            n478 = Delete(path (use dialog)=w1069, error in=w1070) -> (deleted path=w1068:path, error out=w1067:errorcluster)  [unwired: 3 in, 1 out]
          }
        }
        n479 = Move(source path=w1051, error in=w1042, 10:w1043) -> (error out=w1049:errorcluster)  [unwired: 2 in, 2 out]
        n480 = call <vilib>:"Add State(s) to Queue__JKI_lib_State_Machine.vi"("State(s) in (\"\")"=w1064) -> ("States Out"=w1063:string)  [unwired: 14 in]
      }
      frame "Actions: Move All" {
        n481 = Unbundle By Name(w1077) -> ("series path"=w1076:path)
        n482 = local read "New Comics"() -> (w1079:path)
        n483 = property on="New Issues" class="LstBox (strict)"(error in=w1075) -> (error out=w1072:errorcluster, "Item Names"=w1080:string[])  [unwired: 1 in, 1 out]
        n484 = property on="Marvel Issues" class="LstBox (strict)"(error in=w1075) -> (error out=w1073:errorcluster, "Item Names"=w1078:string[])  [unwired: 1 in, 1 out]
        n485 = Merge Errors(w1072, w1073) -> (w1071:errorcluster)
        n486 = for {
          tunnel: w1080 -> [w1090] mode=indexing
          tunnel: w1079 -> [w1089]
          tunnel: w1078 -> [w1088] mode=indexing
          tunnel: w1076 -> [w1087]
          shift-right: [w1084] -> w1074
          shift-left: w1071 -> [w1083]
          n487 = Build Path(base path=w1089, name or relative path=w1090) -> (appended path=w1086:path)
          n488 = Build Path(base path=w1087, name or relative path=w1088) -> (appended path=w1085:path)
          n489 = Move(source path=w1086, error in=w1083, 10:w1085) -> (error out=w1084:errorcluster)  [unwired: 2 in, 2 out]
        }
        n490 = call <vilib>:"Add State(s) to Queue__JKI_lib_State_Machine.vi"("State(s) in (\"\")"=w1082) -> ("States Out"=w1081:string)  [unwired: 14 in]
      }
      frame "Actions: Populate Series" {
        n491 = property on="Folder" class="LstBox (strict)"(error in=w1102) -> (error out=w1101:errorcluster, "Item Names"=w1105:string[], "Value"=w1106:i32)  [unwired: 1 in, 1 out]
        n492 = Unbundle By Name(w1095) -> ("repo path"=w1103:path)
        n493 = Index Array(array=w1105, index=w1106) -> (element=w1104:string)
        n494 = local read "Filter Current"() -> (w1097:bool)
        n495 = Build Path(base path=w1103, name or relative path=w1104) -> (appended path=w1096:path)
        n496 = List Folder(path=w1096, error in=w1101) -> (folder names=w1099:string[], error out=w1098:errorcluster)  [unwired: 2 in, 2 out]
        n497 = case shown="False" w1097 {
          tunnel: [w1113 w1114] -> w1093
          tunnel: w1099 -> [w1113 w1115]
          frame False {
          }
          frame True {
            n498 = for {
              tunnel: w1115 -> [w1117] mode=indexing
              tunnel: [w1117] -> w1114 mode=indexing if=w1116
              n499 = Match Pattern(string=w1117, regular expression=" - present)") -> (offset past match=w1118:i32)  [unwired: 1 in, 3 out]
              n500 = Greater Or Equal To 0?(x=w1118) -> (x >= 0?=w1116:bool)
            }
          }
        }
        n501 = local read "filter string"() -> (w1092:string)
        n502 = for {
          tunnel: w1093 -> [w1111] mode=indexing
          tunnel: [w1111] -> w1094 mode=indexing if=w1110
          tunnel: w1092 -> [w1109]
          n503 = Match Pattern(string=w1111, regular expression=w1109) -> (offset past match=w1112:i32)  [unwired: 1 in, 3 out]
          n504 = Greater Or Equal To 0?(x=w1112) -> (x >= 0?=w1110:bool)
        }
        n505 = property on="Series" class="LstBox (strict)"(error in=w1098, "Item Names"=w1094, "Top Row"=0) -> (error out=w1100:errorcluster)  [unwired: 1 in, 1 out]
        n506 = call <vilib>:"Add State(s) to Queue__JKI_lib_State_Machine.vi"("State(s) in (\"\")"=w1108) -> ("States Out"=w1107:string)  [unwired: 14 in]
      }
      frame "Actions: Build Series Path" {
        n507 = property on="Folder" class="LstBox (strict)"(error in=w1124) -> (error out=w1128:errorcluster, "Item Names"=w1132:string[], "Value"=w1131:i32)  [unwired: 1 in, 1 out]
        n508 = Unbundle By Name(w1121) -> ("repo path"=w1130:path)
        n509 = Index Array(array=w1132, index=w1131) -> (element=w1133:string)
        n510 = property on="Series" class="LstBox (strict)"(error in=w1128) -> (error out=w1123:errorcluster, "Item Names"=w1129:string[], "Value"=w1122:i32)  [unwired: 1 in, 1 out]
        n511 = Build Path(base path=w1130, name or relative path=w1133) -> (appended path=w1127:path)
        n512 = Index Array(array=w1129, index=w1122) -> (element=w1126:string)
        n513 = Build Path(base path=w1127, name or relative path=w1126) -> (appended path=w1125:path)
        n514 = Bundle By Name(cluster=w1121, "series path"=w1125) -> (w1120:T8)
        n515 = call <vilib>:"Add State(s) to Queue__JKI_lib_State_Machine.vi"("State(s) in (\"\")"=w1135) -> ("States Out"=w1134:string)  [unwired: 14 in]
      }
      frame "Actions: Populate Current Issues" {
        w1136 = 0 ("Current Issues")
        n516 = Unbundle By Name(w1143) -> ("series path"=w1142:path)
        n517 = List Folder(path=w1142, pattern="*.cbz", error in=w1141) -> (filenames=w1139:string[], error out=w1138:errorcluster)  [unwired: 1 in, 2 out]
        n518 = property on="Collected Issues" class="LstBox (strict)"(error in=w1138, "Item Names"=w1139, "Value"=w1136, "Top Row"=w1136) -> (error out=w1137:errorcluster)  [unwired: 1 in, 1 out]
        n519 = call <vilib>:"Add State(s) to Queue__JKI_lib_State_Machine.vi"("State(s) in (\"\")"=w1145) -> ("States Out"=w1144:string)  [unwired: 14 in]
      }
      frame "Actions: Populate New Issues" {
        w1146 = 0 ("Current Issues")
        n520 = local read "New Comics"() -> (w1147:path)
        n521 = List Folder(path=w1147, pattern="*.cbz", error in=w1152) -> (filenames=w1150:string[], error out=w1149:errorcluster)  [unwired: 1 in, 2 out]
        n522 = property on="New Issues" class="LstBox (strict)"(error in=w1149, "Item Names"=w1150, "Value"=w1146, "Top Row"=w1146) -> (error out=w1148:errorcluster)  [unwired: 1 in, 1 out]
        n523 = call <vilib>:"Add State(s) to Queue__JKI_lib_State_Machine.vi"("State(s) in (\"\")"=w1155) -> ("States Out"=w1154:string)  [unwired: 14 in]
      }
      frame "Actions: Populate JSON Issues" {
        w1156 = 0 ("Current Issues")
        n524 = Unbundle By Name(w1161) -> ("comic jsons"=w1163:T6[], "json present"=w1162:bool)
        n525 = case shown="True" w1162 {
          tunnel: [_ w1172] -> w1159
          tunnel: w1163 -> [_ w1170]
          tunnel: w1161 -> [w1166 w1169]
          tunnel: [w1166 w1167] -> w1160
          frame False {
          }
          frame True {
            n526 = for {
              tunnel: w1170 -> [w1179] mode=indexing
              tunnel: [w1180] -> w1173 mode=indexing
              n527 = Unbundle By Name(w1179) -> ("title"=w1177:string)
              n528 = call "StandardizeComicTitle.vi"("extention (\"\"=none)"="cbz" ("extention (\"\"=none)"), "title in"=w1177) -> ("title out"=w1180:string)  [unwired: 9 in]
            }
            n529 = call-poly <userlib>:"Sort Array__ogtk.vi"("Array in"=w1173) -> ("Sorted Pointers"=w1171:i32[], "Sorted Array out"=w1172:string[])  [unwired: 9 in]
            n530 = for {
              tunnel: w1171 -> [w1175] mode=indexing
              tunnel: w1170 -> [w1176]
              tunnel: [w1174] -> w1168 mode=indexing
              n531 = Index Array(array=w1176, index=w1175) -> (element=w1174:T6)
            }
            n532 = Bundle By Name(cluster=w1169, "comic jsons"=w1168) -> (w1167:T8)
          }
        }
        n533 = property on="Marvel Issues" class="LstBox (strict)"(error in=w1158, "Item Names"=w1159, "Value"=w1156, "Top Row"=w1156) -> (error out=w1157:errorcluster)  [unwired: 1 in, 1 out]
        n534 = call <vilib>:"Add State(s) to Queue__JKI_lib_State_Machine.vi"("State(s) in (\"\")"=w1165) -> ("States Out"=w1164:string)  [unwired: 14 in]
      }
      frame "Actions: Load JSON" {
        n535 = Unbundle By Name(w1206) -> ("series path"=w1194:path)
        n536 = List Folder(path=w1194, pattern="comics.*.json", error in=w1208) -> (path out=w1197:path, filenames=w1198:string[], error out=w1199:errorcluster)  [unwired: 1 in, 1 out]
        n537 = List Folder(path=w1194, pattern="series.*.json") -> (path out=w1190:path, filenames=w1189:string[], error out=w1188:errorcluster)  [unwired: 2 in, 1 out]
        n538 = Index Array(array=w1198) -> (element=w1204:string)  [unwired: 1 in]
        n539 = Index Array(array=w1189) -> (element=w1191:string)  [unwired: 1 in]
        n540 = Build Path(base path=w1197, name or relative path=w1204) -> (appended path=w1202:path)
        n541 = Build Path(base path=w1190, name or relative path=w1191) -> (appended path=w1192:path)
        n542 = call <vilib>:"Check if File or Folder Exists.vi"("error in (no error)"=w1199, "path"=w1202) -> ("error out"=w1203:errorcluster, "file or folder exists?"=w1200:bool, "dup path"=w1201:path)  [unwired: 7 in]
        n543 = call <vilib>:"Check if File or Folder Exists.vi"("error in (no error)"=w1188, "path"=w1192) -> ("error out"=w1186:errorcluster, "file or folder exists?"=w1187:bool, "dup path"=w1185:path)  [unwired: 7 in]
        n544 = case shown="True" w1200 {
          selector: w1200 -> [w1220 w1222]
          tunnel: [w1221 w1226] -> w1184
          tunnel: [_ w1225] -> w1195
          tunnel: w1203 -> [w1221 w1224]
          tunnel: w1201 -> [_ w1223]
          tunnel: [w1220 w1222] -> w1196
          frame False {
          }
          frame True {
            n545 = Read from Text File(file (use dialog)=w1223, error in=w1224) -> (text=w1229:string, error out=w1228:errorcluster)  [unwired: 2 in, 2 out]
            n546 = call "parse.comics_reply.vi"("error in"=w1228, "string in"=w1229) -> ("error out"=w1226:errorcluster, "data"=w1227:T10)  [unwired: 8 in]
            n547 = Unbundle By Name(w1227) -> ("data.results"=w1225:T6[])
          }
        }
        n548 = case shown="True" w1187 {
          selector: w1187 -> [w1211 w1217]
          tunnel: [w1212 w1215] -> w1183
          tunnel: w1186 -> [w1212 w1219]
          tunnel: w1185 -> [_ w1218]
          tunnel: [w1211 w1217] -> _
          tunnel: [_ w1214] -> w1181
          frame False {
          }
          frame True {
            n549 = Read from Text File(file (use dialog)=w1218, error in=w1219) -> (text=w1213:string, error out=w1216:errorcluster)  [unwired: 2 in, 2 out]
            n550 = call "parse.series.vi"("error in"=w1216, "string in"=w1213) -> ("error out"=w1215:errorcluster, "series json"=w1214:T7)  [unwired: 8 in]
          }
        }
        n551 = Merge Errors(w1184, w1183) -> (w1182:errorcluster)
        n552 = Bundle By Name(cluster=w1206, "json present"=w1196, "comic jsons"=w1195, "series json"=w1181) -> (w1205:T8)
        n553 = call <vilib>:"Add State(s) to Queue__JKI_lib_State_Machine.vi"("State(s) in (\"\")"=w1210) -> ("States Out"=w1209:string)  [unwired: 14 in]
      }
    }
  }
